vi "ME_acquire_19_DeltaForce_Daq_SteppingMode.vi"() -> ()   [LabVIEW 2015]
doc: "Use this template to build a producer/consumer design pattern. Use this template when you need to execute a process, such as data analysis, when a data source, such as a triggered acquisition, produces data at an uneven rate and you need to execute the process when the data becomes available."
uses:
  Mode.ctl
  oxford_driver/Oxford Drivers/BUSGEN.LLB/OxfordAddress.ctl
  <vilib>/Analysis/baseanly.llb/Mean (DBL).vi
  <vilib>/DAQmx/read.llb/DAQmx Read (Analog 1D DBL 1Chan NSamp).vi
  <vilib>/DAQmx/create/channels.llb/DAQmx Create Channel (AI-Voltage-Basic).vi
  <vilib>/DAQmx/configure/timing.llb/DAQmx Timing (Sample Clock).vi
  <vilib>/Utility/file.llb/Write Delimited Spreadsheet (DBL).vi
  <vilib>/DAQmx/miscellaneous.llb/DAQmx Fill In Error Info.vi
  <vilib>/express/express arith-compare/Formula/XNode/ExpressFormulaBlockNode.xnode
  <vilib>/Analysis/NI_AALBase.lvlib
panel:
  out "fractional index or x":dbl
  out "Stepped P(B)":dbl[][](array[numeric])
  out "TimeUp":bool
  out "meanPolarization":dbl format="%0.2f"
  out "Polarization array":dbl[](array[numeric])
  in  "First Offset?":bool
  out "Last2":dbl
  out "Actual2":dbl
  out "Up/Down":bool
  out "T array":dbl[](array[numeric])
  out "Averaged I(T)":dbl[][](array[numeric])
  in  "Averaged P(T)":dbl[][](array[numeric])
  out "remaining elements 2":T1(array[cluster])
  out "Actual mean":dbl format="%0.6f"
  in  "Averaged dt":dbl[][](array[numeric])
  in  "Averaged P(B)":dbl[][](array[numeric])
  out "LockInR":dbl
  out "deltaUaux":dbl
  out "Actual Voltage (V)":dbl caption="Actual AuxV" step=0.1
  in  "Stop":bool
  out "SaveSweep":bool=TRUE
  out "Measurement File_dn":path
  out "Measurement File_up":path
  out "Measurement File_average":path
  out "Actual Polarization":dbl
  in  "Reset IB?":bool
  in  "First?":bool
  in  "Save Period":dbl=1.0
  out "Averaged I(B)":dbl[][](array[numeric])
  out "P(uC/mm^2)":dbl[](array[numeric])
  in  "Sweep":bool
  out "Offset array":dbl[](array[numeric])
  in  "stop 2":bool
  in  "dB":dbl=0.005
  out "appended array":dbl[][](array[numeric])
  out "Actual B Field (T)":dbl
  out "Actual Temperature (K)":dbl
  out "Actual Current (pA)":dbl
  in  "Tab Control":T2(tab)
  in  "dt (K)":dbl=0.1
  in  "Max temperature (K)":dbl=20.0
  in  "Min Temperature (K)":dbl=4.5
  out "P(T)":cluster{dbl[], dbl[]}[](graph)
  out "I(T)":cluster{dbl[], dbl[]}[](graph)
  in  "Set temperature (K)":dbl=4.5
  in  "Temp Ramping Rate (K/min)":dbl=10.0
  in  "Heater Range":enum16{"Off", "Low", "Medium", "High"}(ring)
  in  "Heater On/Off":bool
  out "Setpoint Temperature (K)":dbl
  out "I(T) /Averaged/":cluster{"B array":dbl[], dbl[]}[](graph)
  out "P(T) /Averaged/":cluster{"B array":dbl[], dbl[]}[](graph)
  in  "Stabilization Time (s)":dbl=5.0
  out "I(B) 3":cluster{dbl[], dbl[]}[](graph)
  out "I(B) /Averaged/":cluster{"B array":dbl[], dbl[]}[](graph)
  out "P(B) /Averaged/":cluster{"B array":dbl[], dbl[]}[](graph)
  out "P(B)":cluster{"yi":dbl[], dbl[]}(graph)
  in  "Set Field (T)":dbl
  in  "Go to Set":bool
  in  "Sweep Rate (T/min)":dbl=2.0 format="%.6f"
  in  "Field To Zero":bool
  out "Target Field":dbl
  in  "Min Field (T)":dbl
  in  "Max Field (T)":dbl=0.15
  in  "Threshold B (T)":dbl
  in  "ReOffset":bool=TRUE
  in  "Window (s)":dbl=6.0
  in  "Field Step (T)":dbl=0.01
  in  "Stepping Mode":bool=TRUE
  out "Ready2Step":bool
  in  "Dwell Time (s)":dbl=1.0
  out "B(t)":dbl(graph)
  out "I(t)":dbl(graph)
  out "P(t)":dbl(graph)
  in  "Max count array":i32[](array[numeric])=[2]
  in  "Magnetic Field array (T)":dbl[](array[numeric])=[0.025, 0.05, 0.075, 0.1, 0.125, 0.15, 0.175, 0.2, 0.225, 0.25, 0.275, 0.3]
  in  "T Sweep Rate Array":dbl[](array[numeric])=[10.0, 20.0]
  in  "secs to wait":dbl=180.0
  out "Wait (s)":dbl
  in  "Directory":string
  out "Finished":bool=TRUE
  out "Step Rate":bool
  out "New":bool=TRUE
  in  "Temperature Array":dbl[](array[numeric])=[4.5, 5.0, 6.0, 7.0, 8.0, 9.0, 10.0, 11.0, 12.0]
  in  "Sweep Rate Array":dbl[](array[numeric])=[2.0, 1.0, 0.5, 0.1, 0.05, 9.0, 10.0, 11.0, 12.0]
  in  "Record ALL":bool
  in  "Max Countl":i32
  out "i":i32
  out "j":i32
  out "Step Temp":bool
  in  "FileName":string
  in  "Measure Noise":bool
  in  "Cycles":i32
  in  "maximum value":dbl=10.0 format="%0.2f"
  in  "minimum value":dbl=-10.0 format="%0.2f"
  in  "physical channels":tag="Dev1/ai1"
  out "PSD (pA/Hz^1/2) Peaks Removed":cluster{"f0":dbl, "df":dbl, "magnitude":dbl[]}(graph)
  out "PSD (pA/Hz^1/2)":cluster{"f0":dbl, "df":dbl, "magnitude":dbl[]}(graph)
  out "Current (pA) Filtered":waveform(dbl)(graph)
  out "Current (pA)":dbl[](graph)
  in  "Samples per channel":i32=1000
  in  "Rate":dbl=1000.0 format="%0.2f"
  in  "Cut-Off Frequency":dbl=100.0 caption="Lower Cut-Off"
  in  "Filter On":bool
  in  "Count":i32=60
  in  "Keithley (IV conv) averaging":i32=10
  in  "Lock_in_Amplifier":refnum<visa-resource-name>="GPIB0::5::INSTR"
  out "Dc offset":dbl
  in  "Calibrate":bool
  in  "IV converter":refnum<visa-resource-name>="GPIB0::20::INSTR"
  in  "Magnetic Field":refnum<visa-resource-name>="GPIB0::21::INSTR"
  out "Time Lag":dbl=0.0500025749206543
  in  "Lake Shore":refnum<visa-resource-name>="GPIB0::11::INSTR"
  in  "Temp Refresh (s)":dbl=0.1
  in  "Sampling rate (Hz)":dbl=10.0
  in  "Gain (V/A)":dbl=1000000000.0
  in  "Sample area (mm^2)":dbl=1.0
  out "B_V":cluster{dbl[], "Best Linear Fit":dbl[]}[](graph)=[{[-0.00769241141, -0.00768011662, -0.0029394633, 0.00271952438, 0.00937200583, 0.0154641889, 0.0217080684, 0.0281692221, 0.0344763397, 0.0407091529, 0.0473661569, 0.0541476438, 0.0611164384, 0.0676637725, 0.073937413, 0.0801511723, 0.0863882257, 0.0933787866, 0.0997676928, 0.106163316, 0.113953626, 0.118979018, 0.126030157, 0.132855724, 0.13883398, 0.14631074, 0.153030676, 0.159156864, 0.165801088, 0.17248087, 0.178555009, 0.185285367, 0.192834407, 0.198751051, 0.205413053, 0.212847389, 0.219477697, 0.225574642, 0.232225854, 0.239015189, 0.245675966, 0.252411162, 0.258453848, 0.265211852, 0.271251534, 0.277801221, 0.284008329, 0.291402813, 0.297970768, 0.304082546, 0.310761405, 0.317366634, 0.323522001, 0.330123184, 0.336841279, 0.343557963, 0.349608435, 0.356238003, 0.363590921, 0.370338319, 0.376962983], "Best Linear Fit"=[0.0, 0.0015, 0.0035, 0.0056, 0.0076, 0.0096, 0.0116, 0.0136, 0.0156, 0.0177, 0.0197, 0.0219, 0.0239, 0.0259, 0.0279, 0.0299, 0.032, 0.034, 0.036, 0.038, 0.04, 0.042, 0.0441, 0.046, 0.048, 0.05, 0.052, 0.054, 0.056, 0.058, 0.06, 0.0621, 0.0643, 0.0663, 0.0684, 0.0704, 0.0725, 0.0745, 0.0765, 0.0787, 0.0807, 0.0827, 0.0847, 0.0868, 0.0888, 0.0908, 0.0928, 0.0948, 0.0968, 0.0988, 0.1008, 0.1028, 0.1048, 0.1069, 0.1091, 0.1111, 0.1131, 0.1152, 0.1173, 0.1193, 0.1213]}, {[-0.00769241141, -0.00768011662, -0.0029394633, 0.00271952438, 0.00937200583, 0.0154641889, 0.0217080684, 0.0281692221, 0.0344763397, 0.0407091529, 0.0473661569, 0.0541476438, 0.0611164384, 0.0676637725, 0.073937413, 0.0801511723, 0.0863882257, 0.0933787866, 0.0997676928, 0.106163316, 0.113953626, 0.118979018, 0.126030157, 0.132855724, 0.13883398, 0.14631074, 0.153030676, 0.159156864, 0.165801088, 0.17248087, 0.178555009, 0.185285367, 0.192834407, 0.198751051, 0.205413053, 0.212847389, 0.219477697, 0.225574642, 0.232225854, 0.239015189, 0.245675966, 0.252411162, 0.258453848, 0.265211852, 0.271251534, 0.277801221, 0.284008329, 0.291402813, 0.297970768, 0.304082546, 0.310761405, 0.317366634, 0.323522001, 0.330123184, 0.336841279, 0.343557963, 0.349608435, 0.356238003, 0.363590921, 0.370338319, 0.376962983], "Best Linear Fit"=[0.002353460844818253, 0.002357267374965663, 0.003824997997530172, 0.005577049655813272, 0.007636692089275871, 0.009522863265806463, 0.01145600043639222, 0.013456406815525209, 0.015409122826751182, 0.01733883381400479, 0.019399876452181594, 0.021499459635718428, 0.023657034245452215, 0.025684122519169482, 0.027626473848249778, 0.02955028565017564, 0.03148130942513291, 0.03364562299316916, 0.03562366117513693, 0.037603778974812686, 0.040015698972850115, 0.04157158615356273, 0.04375465501257369, 0.04586788562152819, 0.0477187843918964, 0.050033627699098075, 0.05211415440778254, 0.05401085368533849, 0.056067939569859164, 0.05813603439385595, 0.06001661903361471, 0.06210037244704129, 0.06443759401357516, 0.0662694173922171, 0.06833200743687069, 0.07063371605572277, 0.07268649347515121, 0.0745741389696738, 0.07663338837489471, 0.07873540137051047, 0.08079761214887074, 0.08288286343195213, 0.08475371006132383, 0.08684602281837933, 0.08871593939391825, 0.09074375613756333, 0.09266550866283872, 0.09495487889775463, 0.09698835150804998, 0.09888058937557581, 0.10094839843403076, 0.10299341126621803, 0.10489914451207855, 0.10694290468187984, 0.10902286140750632, 0.11110238128028392, 0.11297563849525552, 0.11502818680688229, 0.1173046879946565, 0.11939371707962458, 0.12144474708765744]}]
  out "V_I":cluster{dbl[], "Best Linear Fit":dbl[]}[](graph)=[{[0.0, 0.012, 0.026, 0.04, 0.054, 0.068, 0.081, 0.096, 0.11, 0.124, 0.138, 0.153, 0.167, 0.18, 0.195, 0.208, 0.223, 0.236, 0.251, 0.265, 0.279, 0.292, 0.306, 0.32, 0.334, 0.348, 0.362, 0.375, 0.389, 0.403, 0.417, 0.432, 0.446, 0.46, 0.475, 0.489, 0.504, 0.517, 0.531, 0.546, 0.56, 0.574, 0.588, 0.602, 0.616, 0.63, 0.644, 0.658, 0.672, 0.685, 0.699, 0.713, 0.727, 0.742, 0.755, 0.77, 0.784, 0.799, 0.814, 0.827, 0.841], "Best Linear Fit"=[-0.00769241141, -0.00768011662, -0.0029394633, 0.00271952438, 0.00937200583, 0.0154641889, 0.0217080684, 0.0281692221, 0.0344763397, 0.0407091529, 0.0473661569, 0.0541476438, 0.0611164384, 0.0676637725, 0.073937413, 0.0801511723, 0.0863882257, 0.0933787866, 0.0997676928, 0.106163316, 0.113953626, 0.118979018, 0.126030157, 0.132855724, 0.13883398, 0.14631074, 0.153030676, 0.159156864, 0.165801088, 0.17248087, 0.178555009, 0.185285367, 0.192834407, 0.198751051, 0.205413053, 0.212847389, 0.219477697, 0.225574642, 0.232225854, 0.239015189, 0.245675966, 0.252411162, 0.258453848, 0.265211852, 0.271251534, 0.277801221, 0.284008329, 0.291402813, 0.297970768, 0.304082546, 0.310761405, 0.317366634, 0.323522001, 0.330123184, 0.336841279, 0.343557963, 0.349608435, 0.356238003, 0.363590921, 0.370338319, 0.376962983]}, {[0.0, 0.012, 0.026, 0.04, 0.054, 0.068, 0.081, 0.096, 0.11, 0.124, 0.138, 0.153, 0.167, 0.18, 0.195, 0.208, 0.223, 0.236, 0.251, 0.265, 0.279, 0.292, 0.306, 0.32, 0.334, 0.348, 0.362, 0.375, 0.389, 0.403, 0.417, 0.432, 0.446, 0.46, 0.475, 0.489, 0.504, 0.517, 0.531, 0.546, 0.56, 0.574, 0.588, 0.602, 0.616, 0.63, 0.644, 0.658, 0.672, 0.685, 0.699, 0.713, 0.727, 0.742, 0.755, 0.77, 0.784, 0.799, 0.814, 0.827, 0.841], "Best Linear Fit"=[-0.015941127780698654, -0.010342478990544012, -0.0038107220686969304, 0.0027210348531501527, 0.009252791774997235, 0.01578454869684432, 0.02184975155284518, 0.028848062540538483, 0.03537981946238557, 0.041911576384232645, 0.048443333306079736, 0.05544164429377303, 0.061973401215620116, 0.06803860407162098, 0.07503691505931429, 0.08110211791531513, 0.08810042890300844, 0.0941656317590093, 0.10116394274670261, 0.1076956996685497, 0.11422745659039678, 0.12029265944639762, 0.1268244163682447, 0.1333561732900918, 0.13988793021193888, 0.14641968713378595, 0.15295144405563305, 0.15901664691163392, 0.165548403833481, 0.1720801607553281, 0.17861191767717516, 0.18561022866486845, 0.19214198558671555, 0.19867374250856262, 0.20567205349625592, 0.212203810418103, 0.2192021214057963, 0.22526732426179719, 0.23179908118364426, 0.23879739217133758, 0.24532914909318465, 0.2518609060150317, 0.2583926629368788, 0.2649244198587259, 0.271456176780573, 0.27798793370242003, 0.28451969062426713, 0.29105144754611423, 0.2975832044679613, 0.3036484073239622, 0.31018016424580924, 0.3167119211676563, 0.3232436780895034, 0.3302419890771967, 0.3363071919331976, 0.3433055029208909, 0.34983725984273795, 0.35683557083043127, 0.36383388181812454, 0.3698990846741254, 0.3764308415959725]}]
  out "B0 (T)":dbl=0.002883352659639724
  out "B/V (T/V)":dbl=0.28933698328911694
  out "I0 (A)":dbl=-0.009969607826625851
  out "V/I (Ohm)":dbl=0.49959372813071373
  in  "Offset?":bool
  in  "Magnet":bool=TRUE
  in  "Ramp":bool=TRUE
  in  "DaQ":bool
  in  "Moving average":i8=10
  in  "Sample Rate":dbl=1000.0
  in  "Number of Samples":i32=100
  in  "Physical Channel":tag="kartya/ai0"
  in  "Min Voltage":dbl=-5.0
  in  "Max Voltage":dbl=5.0
  in  "Terminal Configuration":i32(ring)=-1 items=["default"=-1, "RSE"=10083, "NRSE"=10078, "Differential"=10106, "Pseudodifferential"=12529]
  out "Confirm":bool
  in  "Dwell Time (ms)":u32=1000
  in  "TimeLag?":bool
  in  "Temp/Magnetic Field":bool
  out "index":i8
  out "Read?":bool
  out "Magnetic Field (T)":dbl[](array[numeric])
  out "Reset":bool
  out "Measured Current (pA)":dbl[](array[numeric])
  out "Elapsed Time (s)":dbl[](array[numeric])
  out "Start time":timestamp
  in  "Enum":T3=enum."Process"
  out "B array":dbl[](array[numeric])
  in  "dB (T)":dbl=0.0025
  in  "Counter":i8
  out "L magnet (H)":dbl
  out "R magnet (mOhm)":dbl
  out "Actual Current (R0)":dbl
  out "Actual Field (T)":dbl
  out "Temperature array":dbl[](array[numeric])
  in  "New Measurement File":bool
  out "Measurement File":path
  out "refnum out":refnum<file>
  in  "Measuring":bool
  in  "Measure /Pause":bool
  in  "stop":bool
  # "DeltaForce"
  # "Discrete"
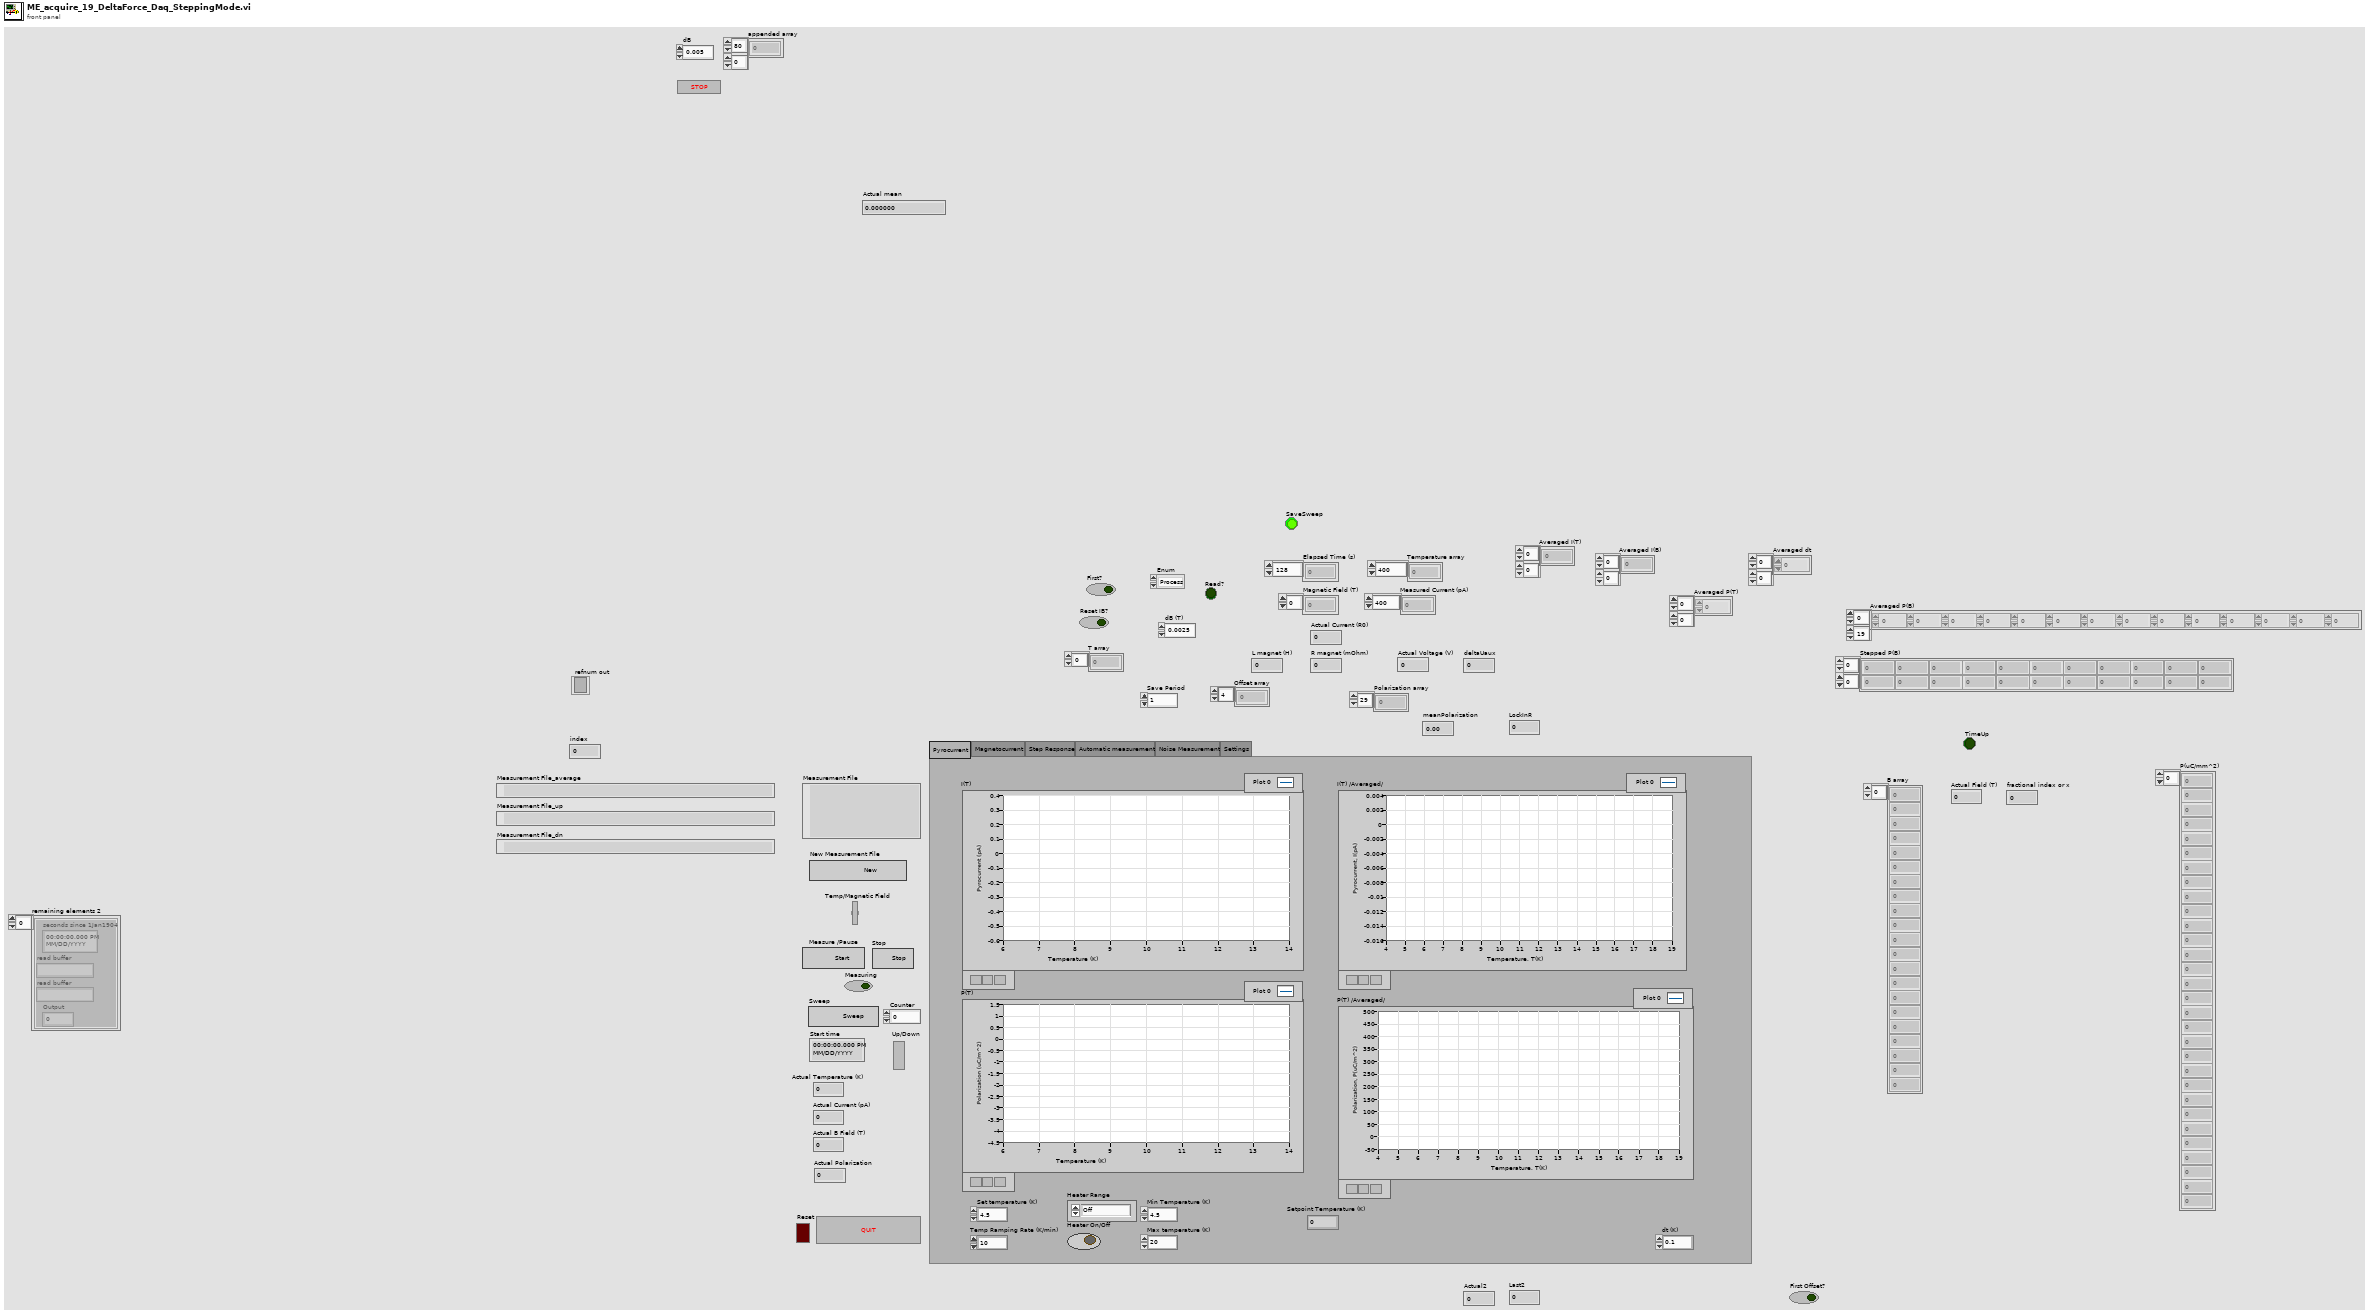
[diagram p1: front panel]
types:
  T1 = cluster{"seconds since 1Jan1904":timestamp, "read buffer":string, "read buffer":string, "Output":dbl}[]
  T2 = enum32{"Pyrocurrent", "Magnetocurrent", "Step Response", "Automatic measurement", "Noise Measurement", "Settings"}
  T3 = typedef "Mode.ctl" = enum16{"Offset", "Process", "Sweep", "StepOxford", "StepDelta", "Plot", "Save", "New", "Return", ""}
  T4 = cluster{"seconds since 1Jan1904":timestamp, "read buffer":string, "read buffer":string, "Output":dbl}
  T5 = enum16{"open", "replace", "create", "open or create", "replace or create", "replace or create with confirmation"}
  T6 = typedef "OxfordAddress.ctl" = cluster{"Com Port":i32, "ISOBUS Address":i32, "GPIB Address":i16, "Communication":enum16{"RS232", "ISOBUS", "GPIB", "Gateway"}}
  T7 = cluster{"B array":dbl[], "Averaged P(B) Out":dbl[]}
  T8 = cluster{"B array":dbl[], "BaselineSubtracted I(B)":dbl[]}
  T9 = cluster{"B array":dbl[], "Averaged P(B) Out":dbl[]}[]
  T10 = cluster{"B array":dbl[], "BaselineSubtracted I(B)":dbl[]}[]
  T11 = cluster{"B array":dbl[], "Averaged P(B)":dbl[]}[]
  T12 = cluster{"T array":dbl[], "Averaged P(T) Out":dbl[]}
  T13 = cluster{"T array":dbl[], "Averaged I(B) out":dbl[]}
  T14 = cluster{"T array":dbl[], "Averaged P(T) Out":dbl[]}[]
  T15 = cluster{"T array":dbl[], "Averaged I(B) out":dbl[]}[]
  T16 = cluster{"V array out (V)":dbl[], "I array out (A)":dbl[]}
  T17 = cluster{"V array out (V)":dbl[], "Best Linear Fit":dbl[]}
  T18 = cluster{"I array out (A)":dbl[], "B array Out":dbl[]}
  T19 = cluster{"I array out (A)":dbl[], "Best Linear Fit 2":dbl[]}
  T20 = cluster{"V array out (V)":dbl[], "Best Linear Fit":dbl[]}[]
  T21 = cluster{"I array out (A)":dbl[], "Best Linear Fit 2":dbl[]}[]
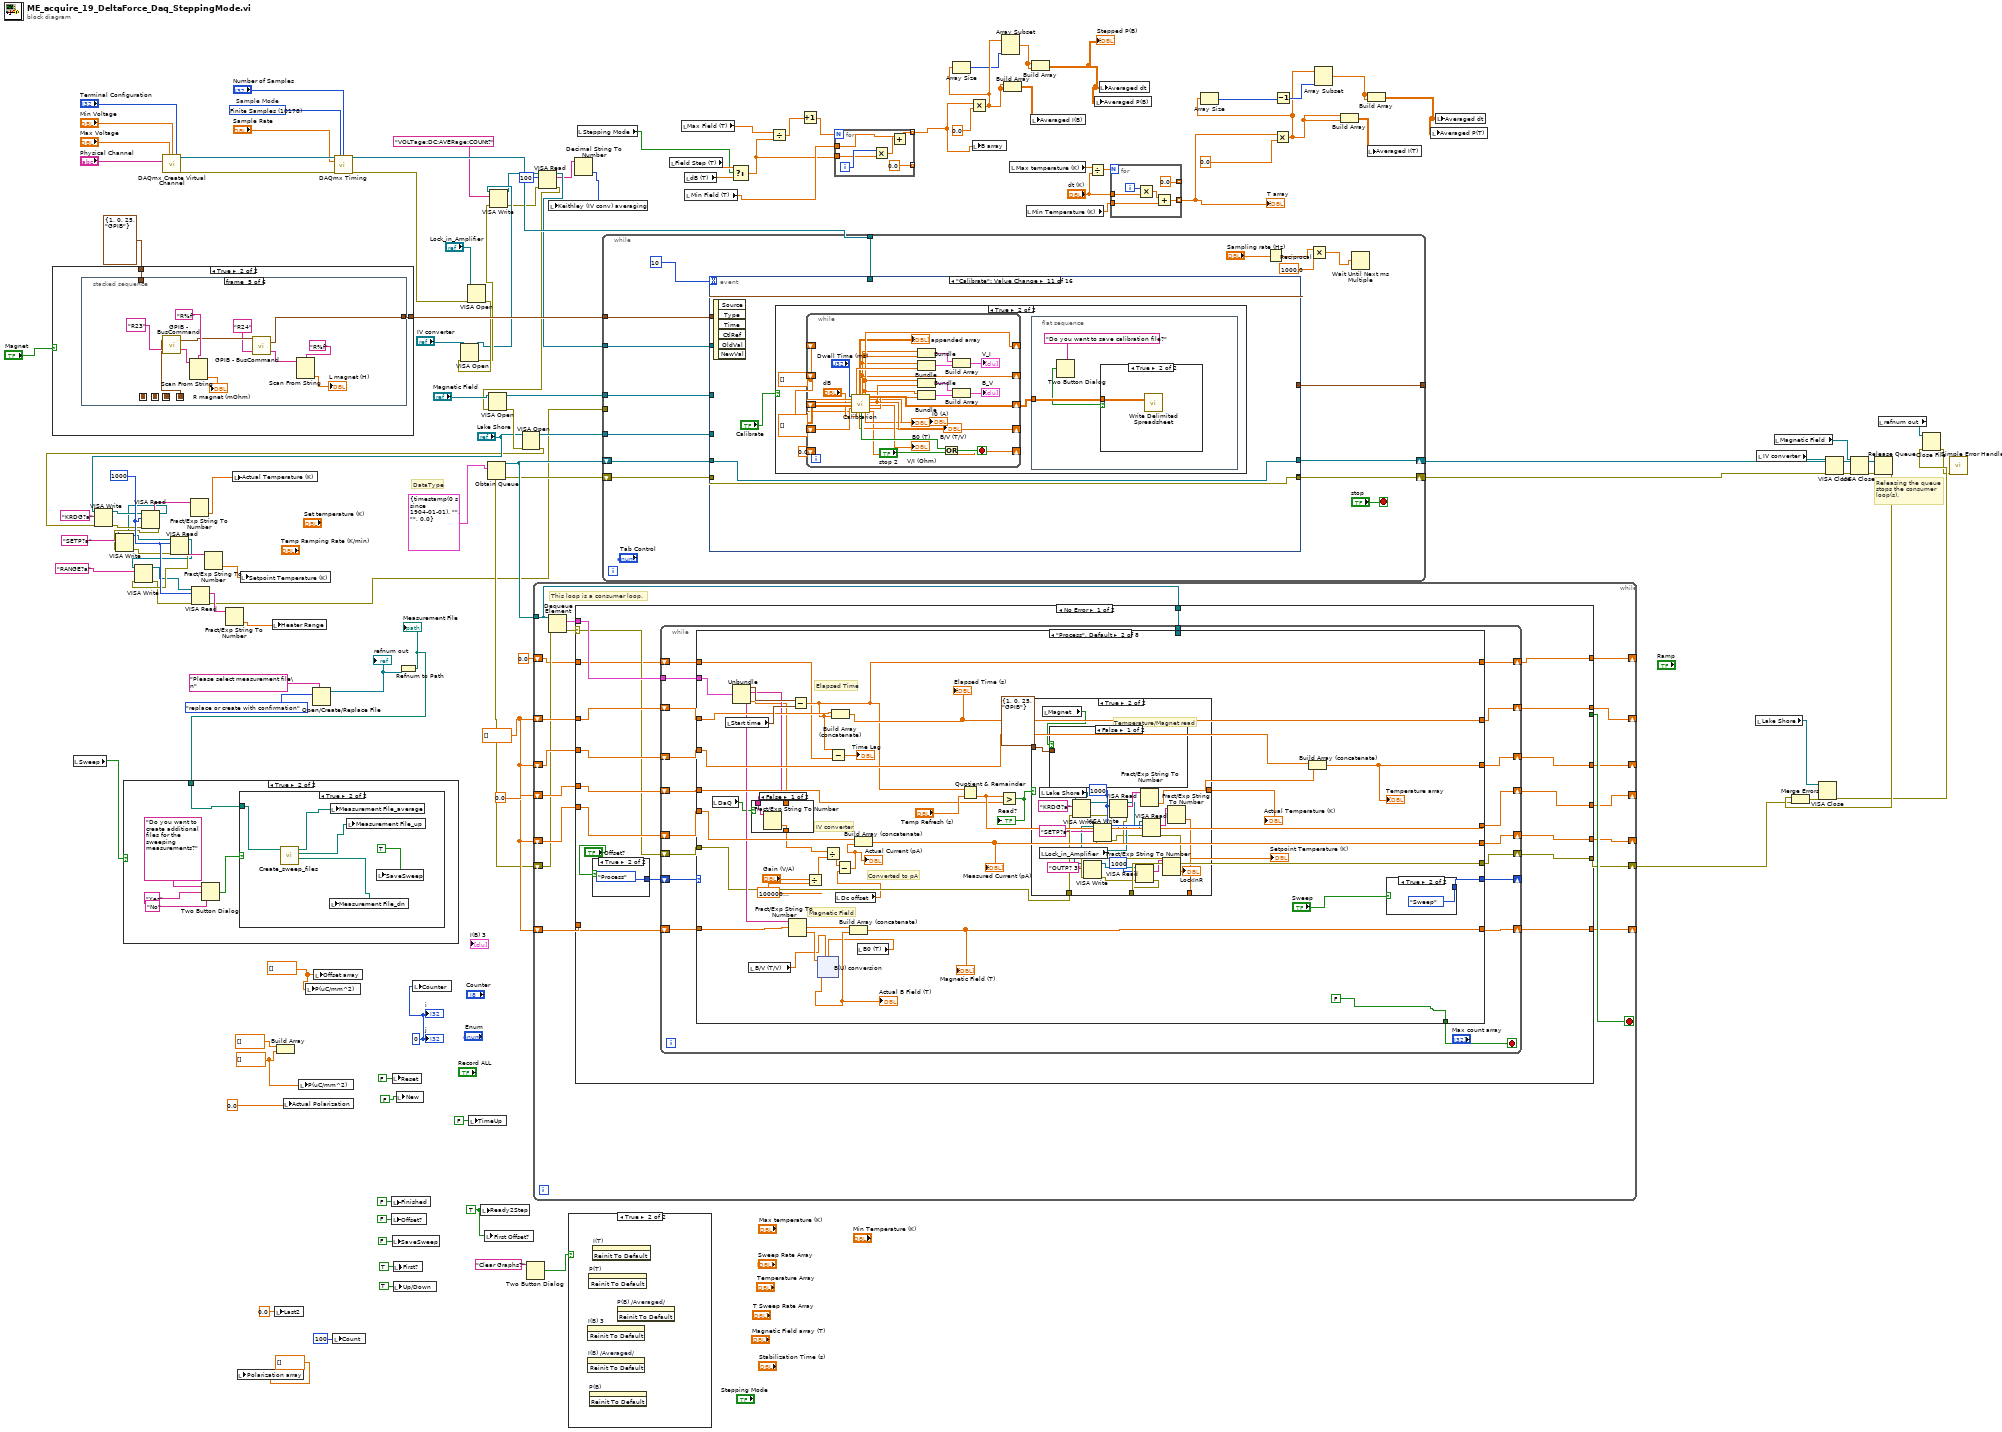
[diagram p0: block diagram]
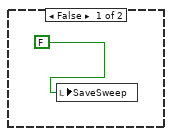
[diagram p4: hidden frame]
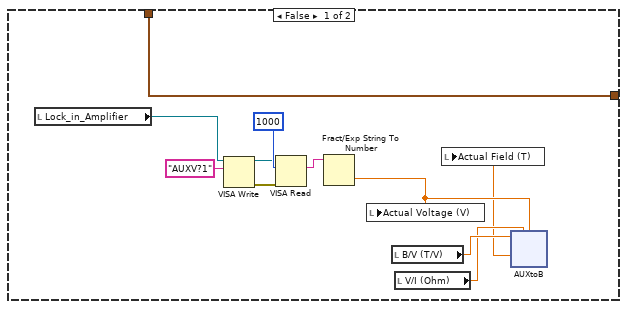
[diagram p5: hidden frame]
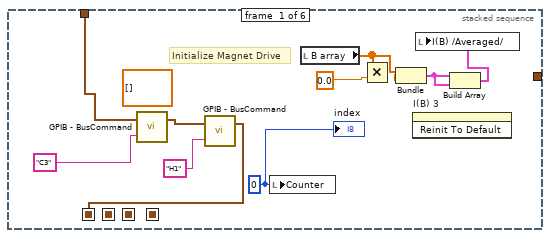
[diagram p6: hidden frame]
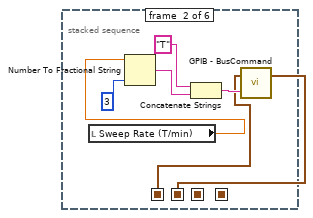
[diagram p7: hidden frame]
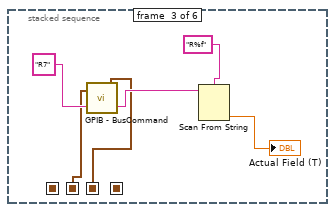
[diagram p8: hidden frame]
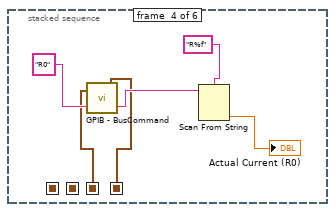
[diagram p9: hidden frame]
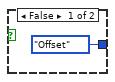
[diagram p11: hidden frame]
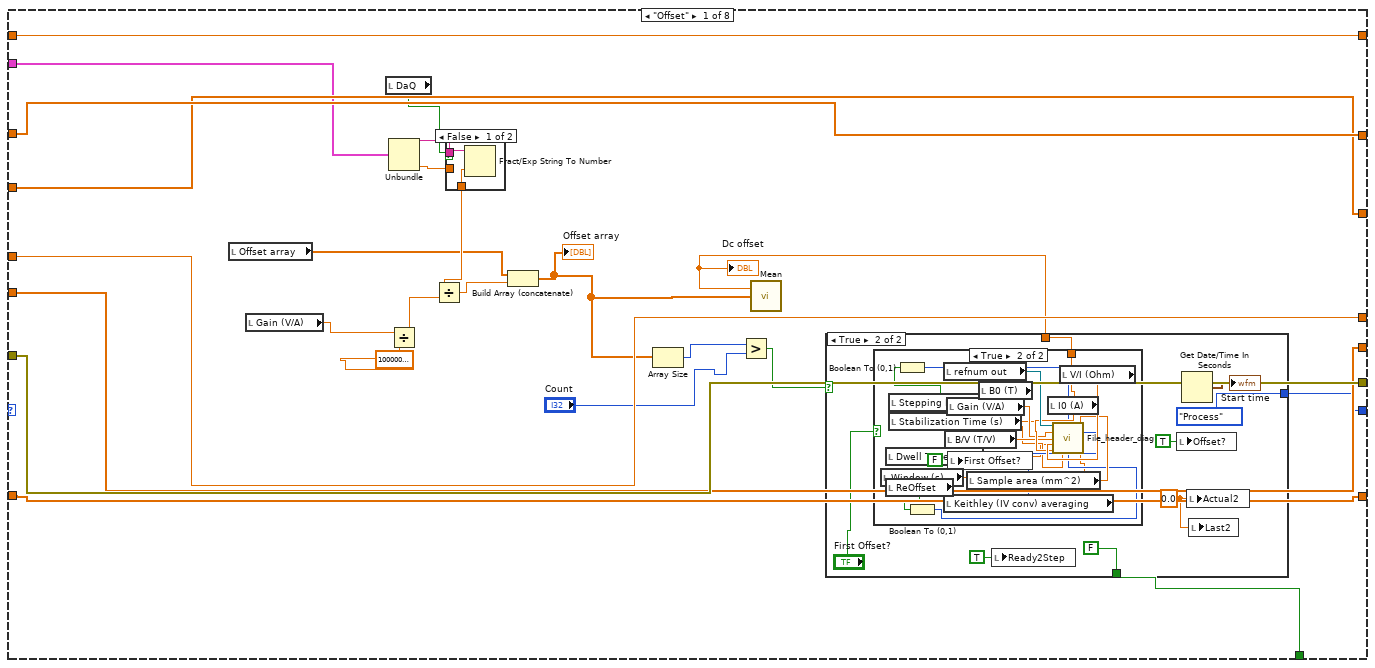
[diagram p12: hidden frame]
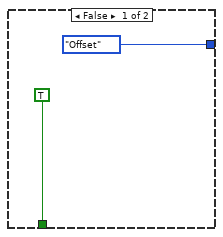
[diagram p14: hidden frame]
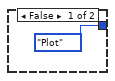
[diagram p17: hidden frame]
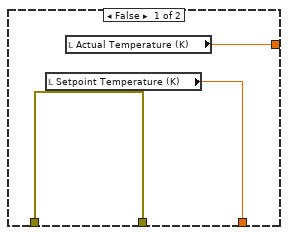
[diagram p18: hidden frame]
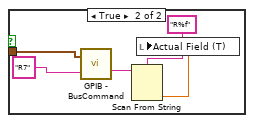
[diagram p19: hidden frame]
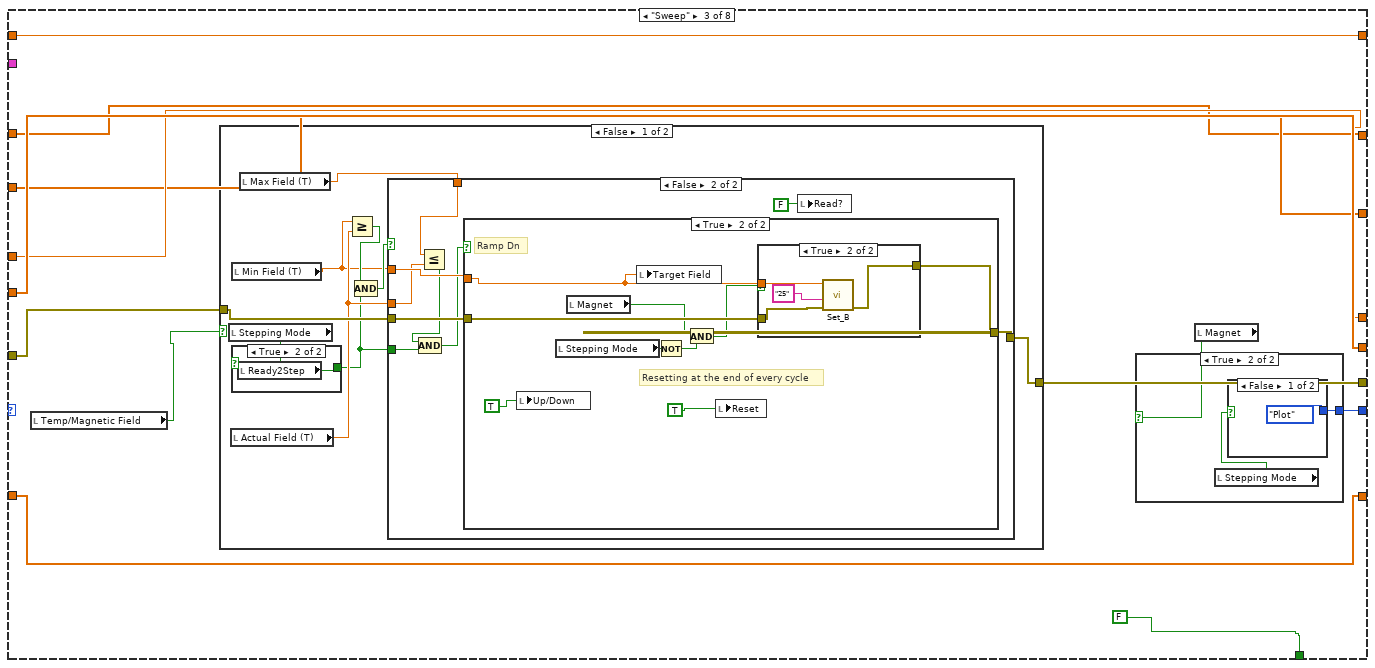
[diagram p20: hidden frame]
diagram:
  w13 = TRUE ("Ready2Step")
  w48 = 10178 items=["Finite Samples"=10178, "Continuous Samples"=10123, "Hardware Timed Single Point"=12522]  # Sample Mode
  w72 = u32 1000 ("byte count")
  w83 = 0 ("j")
  w80 = dbl[] []
  w95 = dbl[] []
  w101 = dbl[] []
  # "DataType"
  # "Releasing the queue stops the consumer loop(s)."
  n1 = case shown="True" "Magnet" {
    tunnel: T6 {"Com Port"=1, "ISOBUS Address"=0, "GPIB Address"=25, "Communication"=enum."GPIB"} ("Address") -> [w135 w149]
    tunnel: [w135 w148] -> w107
    frame False {
      n2 = local read "Lock_in_Amplifier"() -> (w129:refnum<visa-resource-name>)
      n3 = VISA Write(VISA resource name=w129, write buffer="AUXV?1") -> (VISA resource name out=w130:refnum<visa-resource-name>, error out=w134:errorcluster)  [unwired: 1 in, 1 out]
      n4 = VISA Read(VISA resource name=w130, byte count=u32 1000, error in (no error)=w134) -> (read buffer=w133:string)  [unwired: 3 out]
      n5 = Fract/Exp String To Number(string=w133) -> (number=w126:dbl)  [unwired: 3 in, 1 out]
      n6 = local write "Actual Voltage (V)"(w126) -> ()
      n7 = local read "B/V (T/V)"() -> (w128:dbl)
      n8 = local read "V/I (Ohm)"() -> (w127:dbl)
      n9 = xnode "AUXtoB"("BpV"=w128, "Rm"=w127, "Aux"=w126) -> ("Result"=w125:dbl)  [unwired: 1 in, 1 out]
      n10 = local write "Actual Field (T)"(w125) -> ()
    }
    frame True {
      n11 = stacked-sequence {
        seq-local: [w157 _ _ _ _ _] -> [_ w162 _ _ _ _]
        seq-local: [_ w161 _ _ _ _] -> [_ _ w169 _ _ _]
        seq-local: [_ _ w168 _ _ _] -> [_ _ _ w175 _ _]
        seq-local: [_ _ _ w174 _ _] -> [_ _ _ _ w186 _]
        tunnel: w149 -> [w159 _ _ _ _ _]
        tunnel: [_ _ _ _ w184 _] -> w148
        frame #0 {
          (unwired) dbl[][] []
          w155 = i8 0 ("Counter")
          # "Initialize Magnet Drive"
          n12 = call "GPIB - BusCommand.vi"("Command"="C3", "Address"=w159) -> ("Address(thru)"=w158:T6)  [unwired: 1 out]
          n13 = call "GPIB - BusCommand.vi"("Command"="H1", "Address"=w158) -> ("Address(thru)"=w157:T6)  [unwired: 1 out]
          n14 = local write "Counter"(w155) -> ()
          n15 = local read "B array"() -> (w153:dbl[])
          n16 = Multiply(x=w153, y=0.0) -> (x*y=w152:dbl[])
          n17 = Bundle("B array"=w153, w152) -> (w151:cluster{"B array":dbl[], dbl[]})  [unwired: 1 in]
          n18 = invoke on="I(B) 3" class="XYGraph (strict)" method="Reinit To Default"() -> ()  [unwired: 3 in, 3 out]
          n19 = Build Array(w151, w151) -> (w150:cluster{"B array":dbl[], dbl[]}[])
          n20 = local write "I(B) /Averaged/"(w150) -> ()
          "index" <- w155
        }
        frame #1 {
          n21 = local read "Sweep Rate (T/min)"() -> (w163:dbl)
          n22 = Number To Fractional String(number=w163, precision (6)=i16 3) -> (F-format string=w165:string)  [unwired: 2 in]
          n23 = Concatenate Strings("T" ("format string"), w165) -> (w164:string)
          n24 = call "GPIB - BusCommand.vi"("Command"=w164, "Address"=w162) -> ("Address(thru)"=w161:T6)  [unwired: 1 out]
        }
        frame #2 {
          n25 = call "GPIB - BusCommand.vi"("Command"="R7" ("format string"), "Address"=w169) -> ("Reply"=w173:string, "Address(thru)"=w168:T6)
          n26 = Scan From String(format string="R%f" ("remaining string"), input string=w173) -> (output 1=→"Actual Field (T)":dbl)  [unwired: 3 in, 3 out]
        }
        frame #3 {
          n27 = call "GPIB - BusCommand.vi"("Command"="R0" ("format string"), "Address"=w175) -> ("Reply"=w179:string, "Address(thru)"=w174:T6)
          n28 = Scan From String(format string="R%f" ("remaining string"), input string=w179) -> (output 1=→"Actual Current (R0)":dbl)  [unwired: 3 in, 3 out]
        }
        frame #4 {
          n29 = call "GPIB - BusCommand.vi"("Command"="R23" ("format string"), "Address"=w186) -> ("Reply"=w190:string, "Address(thru)"=w185:T6)
          n30 = Scan From String(format string="R%f" ("remaining string"), input string=w190) -> (output 1=→"R magnet (mOhm)":dbl)  [unwired: 3 in, 3 out]
          n31 = call "GPIB - BusCommand.vi"("Command"="R24" ("format string"), "Address"=w185) -> ("Reply"=w182:string, "Address(thru)"=w184:T6)
          n32 = Scan From String(format string="R%f" ("remaining string"), input string=w182) -> (output 1=→"L magnet (H)":dbl)  [unwired: 3 in, 3 out]
        }
        frame #5 {
        }
      }
    }
  }
  n33 = local read "Sweep"() -> (w88:bool)
  n34 = call-poly <vilib>:"DAQmx Create Virtual Channel.vi"("maximum value"="Max Voltage", "minimum value"="Min Voltage", "input terminal configuration"="Terminal Configuration", "physical channels"="Physical Channel") -> ("task out"=w46:refnum<k21>, "error out"=w47:errorcluster)  [unwired: 10 in]
  n35 = local write "Polarization array"(dbl[] [] ("Polarization array")) -> ()
  n36 = local write "Last2"(0.0 ("Last2")) -> ()
  n37 = Build Array(dbl[] [], w80) -> ()  [unwired: 1 out]
  n38 = local write "Actual Polarization"(0.0 ("Actual Polarization")) -> ()
  n39 = local write "P(uC/mm^2)"(w80) -> ()
  n40 = local write "P(uC/mm^2)"(w95) -> ()
  n41 = Open/Create/Replace File(prompt="Please select measurement file\n", operation (0:open)=T5."replace or create with confirmation") -> (refnum out=w104:refnum<file>)  [unwired: 4 in, 2 out]
  "refnum out" <- w104
  n42 = local write "Offset array"(w95) -> ()
  n43 = local write "Count"(100 ("Count")) -> ()
  n44 = call-poly <vilib>:"DAQmx Timing.vi"("task/channels in"=w46, "sample mode"=w48, "samples per channel"="Number of Samples", "rate"="Sample Rate", "error in"=w47) -> ("task out"=w38:refnum<k21>, "error out"=w39:errorcluster)  [unwired: 9 in]
  n45 = local write "Finished"(FALSE ("Finished")) -> ()
  n46 = local write "Offset?"(FALSE ("Offset?")) -> ()
  n47 = local write "Reset"(FALSE ("Reset")) -> ()
  n48 = local write "SaveSweep"(FALSE ("SaveSweep")) -> ()
  n49 = local write "First?"(TRUE ("First?")) -> ()
  n50 = local write "Up/Down"(TRUE ("Up/Down")) -> ()
  n51 = local write "New"(FALSE ("New")) -> ()
  n52 = Refnum to Path(1:w104) -> (0:w87:path)
  "Measurement File" <- w87
  n53 = case shown="True" w88 {
    tunnel: w87 -> [_ w191]
    frame False {
    }
    frame True {
      n54 = Two Button Dialog(message="Do you want to create additional files for the sweeping measurements?" ("string"), 1:"No" ("F button name (\"Cancel\")"), 2:"Yes" ("T button name (\"OK\")")) -> (T button?=w193:bool)
      n55 = case shown="True" w193 {
        tunnel: w191 -> [_ w201]
        frame False {
          n56 = local write "SaveSweep"(FALSE ("SaveSweep")) -> ()
        }
        frame True {
          n57 = call "Create_sweep_files.vi"("Measurement File"=w201) -> ("Path 3"=w198:path, "Path 2"=w199:path, "Path"=w200:path)  [unwired: 8 in]
          n58 = local write "Measurement File_dn"(w198) -> ()
          n59 = local write "Measurement File_average"(w200) -> ()
          n60 = local write "Measurement File_up"(w199) -> ()
          n61 = local write "SaveSweep"(TRUE) -> ()
        }
      }
    }
  }
  n62 = local write "Counter"(w83) -> ()
  n63 = VISA Open(error in (no error)=w39, VISA resource name="Lock_in_Amplifier") -> (error out=w55:errorcluster)  [unwired: 3 in, 1 out]
  n64 = VISA Open(error in (no error)=w55, VISA resource name="IV converter") -> (VISA resource name=w35:refnum<visa-resource-name>, error out=w36:errorcluster)  [unwired: 3 in]
  n65 = local write "TimeUp"(FALSE ("TimeUp")) -> ()
  n66 = local write "Ready2Step"(w13) -> ()
  n67 = local write "First Offset?"(w13) -> ()
  n68 = Obtain Queue(element data type=T4 {"seconds since 1Jan1904"=timestamp(0 s since 1904-01-01), "read buffer"="", "read buffer"="", "Output"=0.0} ("output cluster")) -> (queue out=w124:refnum<queue>, error out=w99:errorcluster)  [unwired: 4 in, 1 out]
  n69 = VISA Write(VISA resource name=w35, write buffer="VOLTage:DC:AVERage:COUNt?", error in (no error)=w36) -> (VISA resource name out=w31:refnum<visa-resource-name>, error out=w33:errorcluster)  [unwired: 1 out]
  n70 = Two Button Dialog(message="Clear Graphs?") -> (T button?=w82:bool)  [unwired: 2 in]
  n71 = while {
    tunnel: w124 -> [w202]
    shift-right: [w215] -> _
    shift-left: w101 -> [w214]
    shift-right: [w213] -> _
    shift-left: w101 -> [w212]
    shift-right: [w211] -> _
    shift-left: w101 -> [w210]
    shift-right: [w209] -> _
    shift-left: 0.0 -> [w208]
    shift-right: [w207] -> _
    shift-left: w101 -> [w206]
    shift-right: [w216] -> w112
    shift-left: w99 -> [w205]
    shift-right: [w204] -> _
    shift-left: 0.0 -> [w203]
    stop <- w217 stop-if-true
    # "This loop is a consumer loop."
    n72 = Dequeue Element(queue=w202, error in (no error)=w205) -> (element=w218:T4, error out=w219:errorcluster)  [unwired: 1 in, 2 out]
    n73 = case shown="No Error" w219 {
      selector: w219 -> [w225 w1221]
      tunnel: w218 -> [w236 _]
      tunnel: [_ TRUE] -> w217
      tunnel: [w224 w1221] -> w216
      tunnel: [w235 w1220] -> w215
      tunnel: w214 -> [w234 w1220]
      tunnel: [w233 w1217] -> w213
      tunnel: w212 -> [w232 w1217]
      tunnel: [w231 w1216] -> w211
      tunnel: w210 -> [w230 w1216]
      tunnel: [w229 w1218] -> w209
      tunnel: w208 -> [w228 w1218]
      tunnel: [w227 w1219] -> w207
      tunnel: w206 -> [w226 w1219]
      tunnel: [w223 w1215] -> w204
      tunnel: w203 -> [w222 w1215]
      tunnel: w202 -> [w220 _]
      frame No Error {
        n74 = case shown="True" "Offset?" {
          tunnel: [Mode."Offset" ("Enum") Mode."Process" ("Enum")] -> w237
          frame False {
          }
          frame True {
          }
        }
        n75 = while {
          shift-right: [w246] -> _
          shift-left: w237 -> [w258]
          tunnel: w236 -> [w257]
          shift-right: [w256] -> w235
          shift-left: w234 -> [w255]
          shift-right: [w248] -> w227
          shift-left: w226 -> [w247]
          shift-right: [w250] -> w229
          shift-left: w228 -> [w249]
          shift-right: [w254] -> w233
          shift-left: w232 -> [w253]
          shift-right: [w244] -> w224
          shift-left: w225 -> [w245]
          shift-right: [w252] -> w231
          shift-left: w230 -> [w251]
          shift-right: [w242] -> w223
          shift-left: w222 -> [w241]
          tunnel: w220 -> [w240]
          stop <- w243 stop-if-true
          n76 = case shown="\"Process\", Default" w258 {
            selector: w258 -> [_ _ _ _ _ _ _ w1208]
            tunnel: w257 -> [w276 w351 _ _ _ _ _ _]
            tunnel: [w282 w348 w409 w558 w702 w820 w984 w1213] -> w256
            tunnel: w255 -> [w282 w341 w409 w558 w702 w816 w984 w1213]
            tunnel: [w277 w347 w412 w555 w704 w822 w982 w1210] -> w254
            tunnel: w253 -> [w277 w346 w412 w555 w704 w817 w982 w1210]
            tunnel: [w278 w345 w414 w554 w699 w823 w980 w1207] -> w252
            tunnel: w251 -> [w278 w344 w414 w554 w699 w818 w980 w1207]
            tunnel: [w280 w340 w411 w556 w700 w826 0.0 w1211] -> w250
            tunnel: w249 -> [w280 w339 w411 w556 w700 w826 _ w1211]
            tunnel: [w281 w336 w410 w557 w701 w821 w983 w1212] -> w248
            tunnel: w247 -> [w281 w337 w410 w557 w701 w819 w983 w1212]
            tunnel: [w266 w334 w407 Mode."Plot" ("Enum") Mode."Save" ("Enum") w827 Mode."Return" ("Enum") w1208] -> w246
            tunnel: w245 -> [w279 w332 w416 w552 w706 w825 w976 w1209]
            tunnel: [w279 w331 w415 w551 w706 w825 w975 w1209] -> w244
            tunnel: [w262 FALSE FALSE FALSE FALSE w814 TRUE TRUE] -> w243
            tunnel: [w265 w328 w408 w549 w703 w824 0.0 w1214] -> w242
            tunnel: w241 -> [w265 w327 w408 w549 w703 w824 _ w1214]
            tunnel: w240 -> [_ _ _ _ _ _ w974 _]
            frame "Offset" {
              n77 = local read "Offset array"() -> (w270:dbl[])
              n78 = local read "Gain (V/A)"() -> (w274:dbl)
              n79 = local read "DaQ"() -> (w261:bool)
              n80 = Unbundle(w276) -> ("read buffer"=w264:string, "Output"=w260:dbl)  [unwired: 2 out]
              n81 = Divide(x=w274, y=1000000000000.0) -> (x/y=w272:dbl)
              n82 = case shown="False" w261 {
                tunnel: [w284 w285] -> w275
                tunnel: w264 -> [w283 _]
                tunnel: w260 -> [_ w285]
                frame False {
                  n83 = Fract/Exp String To Number(string=w283) -> (number=w284:dbl)  [unwired: 3 in, 1 out]
                }
                frame True {
                }
              }
              n84 = Divide(x=w275, y=w272) -> (x/y=w271:dbl)
              n85 = Build Array (concatenate)(w270, w271) -> (w267:dbl[])
              "Offset array" <- w267
              n86 = Array Size(array=w267) -> (size(s)=w269:i32)
              n87 = Greater?(x=w269, y="Count") -> (0:w268:bool)
              n88 = call-poly <vilib>:"Mean.vi"("X"=w267) -> ("mean"=w263:dbl)  [unwired: 1 out]
              "Dc offset" <- w263
              n89 = case shown="True" w268 {
                tunnel: [Mode."Offset" ("Enum") Mode."Process" ("Enum")] -> w266
                tunnel: w263 -> [_ w293]
                tunnel: [TRUE FALSE] -> w262
                frame False {
                }
                frame True {
                  w289 = 0.0 ("Actual2")
                  n90 = case shown="True" "First Offset?" {
                    tunnel: w293 -> [_ w307]
                    frame False {
                    }
                    frame True {
                      n91 = local read "Window (s)"() -> (w297:dbl)
                      n92 = local read "Dwell Time (s)"() -> (w296:dbl)
                      n93 = local read "ReOffset"() -> (w301:bool)
                      n94 = local read "Stepping Mode"() -> (w304:bool)
                      n95 = local read "Stabilization Time (s)"() -> (w298:dbl)
                      n96 = Boolean To (0,1)(Boolean=w304) -> (0, 1=w303:i16)
                      n97 = Boolean To (0,1)(Boolean=w301) -> (0, 1=w300:i16)
                      n98 = local read "refnum out"() -> (w312:refnum<file>)
                      n99 = local read "Keithley (IV conv) averaging"() -> (w306:i32)
                      n100 = local read "B/V (T/V)"() -> (w308:dbl)
                      n101 = local read "Gain (V/A)"() -> (w309:dbl)
                      n102 = local write "First Offset?"(FALSE ("First Offset?")) -> ()
                      n103 = local read "Sample area (mm^2)"() -> (w305:dbl)
                      n104 = local read "B0 (T)"() -> (w299:dbl)
                      n105 = local read "I0 (A)"() -> (w310:dbl)
                      n106 = local read "V/I (Ohm)"() -> (w311:dbl)
                      n107 = call "File_header_diag.vi"("Byte Stream File in"=w312, "B/V"=w308, "SteppingMode"=w303, "OFFSET"=w307, "Sample area"=w305, "Gain"=w309, "Averaging"=w306, "V/I"=w311, "DwellTime"=w296, "I0"=w310, "B0"=w299, "Reoffset"=w300, "Stabilization time"=w298, "Window"=w297) -> ()  [unwired: 2 in]
                    }
                  }
                  n108 = local write "Ready2Step"(TRUE ("Ready2Step")) -> ()
                  n109 = local write "Offset?"(TRUE ("Offset?")) -> ()
                  n110 = Get Date/Time In Seconds() -> (seconds since 1Jan1904=→"Start time":timestamp)
                  n111 = local write "Actual2"(w289) -> ()
                  n112 = local write "Last2"(w289) -> ()
                }
              }
            }
            frame "Process", Default {
              # "Converted to pA"
              # "Magnetic Field"
              # "IV converter"
              # "Elapsed Time"
              n113 = local read "DaQ"() -> (w315:bool)
              n114 = local read "Start time"() -> (w349:timestamp)
              n115 = Unbundle(w351) -> ("seconds since 1Jan1904"=w350:timestamp, "read buffer"=w316:string, "read buffer"=w333:string, "Output"=w313:dbl)
              n116 = local read "B/V (T/V)"() -> (w323:dbl)
              n117 = case shown="False" w315 {
                tunnel: w316 -> [w355 _]
                tunnel: [w354 w356] -> w314
                tunnel: w313 -> [_ w356]
                frame False {
                  n118 = Fract/Exp String To Number(string=w355) -> (number=w354:dbl)  [unwired: 3 in, 1 out]
                }
                frame True {
                }
              }
              n119 = Fract/Exp String To Number(string=w333) -> (number=w343:dbl)  [unwired: 3 in, 1 out]
              n120 = Subtract(x=w350, y=w349) -> (x-y=w328:dbl)
              n121 = Divide(x="Gain (V/A)", y=1000000000000.0) -> (x/y=w326:dbl)
              n122 = Divide(x=w314, y=w326) -> (x/y=w321:dbl)
              n123 = Subtract(x=w328, y=w327) -> (x-y=→"Time Lag":dbl)
              n124 = Build Array (concatenate)(w341, w328) -> (w348:dbl[])
              "Elapsed Time (s)" <- w348
              n125 = local read "Dc offset"() -> (w319:dbl)
              n126 = Subtract(x=w321, y=w319) -> (x-y=w320:dbl)
              "Actual Current (pA)" <- w320
              n127 = Build Array (concatenate)(w346, w320) -> (w347:dbl[])
              "Measured Current (pA)" <- w347
              n128 = local read "B0 (T)"() -> (w322:dbl)
              n129 = xnode "B(U) conversion"("V"=w343, "BpV"=w323, "B0"=w322) -> ("Result"=w342:dbl)  [unwired: 1 in, 1 out]
              "Actual B Field (T)" <- w342
              n130 = Build Array (concatenate)(w344, w342) -> (w345:dbl[])
              "Magnetic Field (T)" <- w345
              n131 = Quotient & Remainder(x=w328, y="Temp Refresh (s)") -> (floor(x/y)=w340:dbl)  [unwired: 1 out]
              n132 = Greater?(x=w340, y=w339) -> (0:w338:bool)
              "Read?" <- w338
              n133 = case shown="True" w338 {
                tunnel: [w360 w385] -> w335
                tunnel: w332 -> [w361 w384]
                tunnel: [w361 w364] -> w331
                tunnel: T6 {"Com Port"=1, "ISOBUS Address"=0, "GPIB Address"=25, "Communication"=enum."GPIB"} ("Address") -> [_ w383]
                tunnel: [w359 w379] -> w317
                frame False {
                  n134 = local read "Setpoint Temperature (K)"() -> (w359:dbl)
                  n135 = local read "Actual Temperature (K)"() -> (w360:dbl)
                }
                frame True {
                  w380 = u32 1000 ("byte count")
                  # "Temperature/Magnet read"
                  n136 = local read "Lock_in_Amplifier"() -> (w368:refnum<visa-resource-name>)
                  n137 = local read "Lake Shore"() -> (w382:refnum<visa-resource-name>)
                  n138 = local read "Magnet"() -> (w371:bool)
                  n139 = case shown="False" w371 {
                    tunnel: w383 -> [_ w389]
                    frame False {
                    }
                    frame True {
                      n140 = call "GPIB - BusCommand.vi"("Command"="R7" ("format string"), "Address"=w389) -> ("Reply"=w390:string)  [unwired: 1 out]
                      n141 = Scan From String(format string="R%f" ("remaining string"), input string=w390) -> (output 1=w388:dbl)  [unwired: 3 in, 3 out]
                      n142 = local write "Actual Field (T)"(w388) -> ()
                    }
                  }
                  n143 = VISA Write(VISA resource name=w382, write buffer="KRDG?a", error in (no error)=w384) -> (VISA resource name out=w378:refnum<visa-resource-name>, error out=w376:errorcluster)  [unwired: 1 out]
                  n144 = VISA Read(VISA resource name=w378, byte count=w380, error in (no error)=w376) -> (VISA resource name out=w377:refnum<visa-resource-name>, read buffer=w386:string, error out=w375:errorcluster)  [unwired: 1 out]
                  n145 = VISA Write(VISA resource name=w377, write buffer="SETP?a", error in (no error)=w375) -> (VISA resource name out=w373:refnum<visa-resource-name>, error out=w374:errorcluster)  [unwired: 1 out]
                  n146 = Fract/Exp String To Number(string=w386) -> (number=w385:dbl)  [unwired: 3 in, 1 out]
                  n147 = VISA Read(VISA resource name=w373, byte count=w380, error in (no error)=w374) -> (read buffer=w372:string, error out=w370:errorcluster)  [unwired: 2 out]
                  n148 = VISA Write(VISA resource name=w368, write buffer="OUTP? 3", error in (no error)=w370) -> (VISA resource name out=w367:refnum<visa-resource-name>, error out=w369:errorcluster)  [unwired: 1 out]
                  n149 = VISA Read(VISA resource name=w367, byte count=u32 1000, error in (no error)=w369) -> (read buffer=w363:string, error out=w364:errorcluster)  [unwired: 2 out]
                  n150 = Fract/Exp String To Number(string=w363) -> (number=→"LockInR":dbl)  [unwired: 3 in, 1 out]
                  n151 = Fract/Exp String To Number(string=w372) -> (number=w379:dbl)  [unwired: 3 in, 1 out]
                }
              }
              "Actual Temperature (K)" <- w335
              "Setpoint Temperature (K)" <- w317
              n152 = Build Array (concatenate)(w337, w335) -> (w336:dbl[])
              "Temperature array" <- w336
              n153 = case shown="True" "Sweep" {
                tunnel: [Mode."Plot" ("Enum") Mode."Sweep" ("Enum")] -> w334
                frame False {
                }
                frame True {
                }
              }
            }
            frame "Sweep" {
              n154 = local read "Temp/Magnetic Field"() -> (w406:bool)
              n155 = case shown="False" w406 {
                tunnel: w416 -> [w429 w496]
                tunnel: [w428 w495] -> w415
                frame False {
                  n156 = local read "Stepping Mode"() -> (w423:bool)
                  n157 = local read "Actual Field (T)"() -> (w425:dbl)
                  n158 = local read "Min Field (T)"() -> (w424:dbl)
                  n159 = case shown="True" w423 {
                    tunnel: [w431 w432] -> w422
                    frame False {
                      n160 = local read "Read?"() -> (w431:bool)
                    }
                    frame True {
                      n161 = local read "Ready2Step"() -> (w432:bool)
                    }
                  }
                  n162 = local read "Max Field (T)"() -> (w430:dbl)
                  n163 = Greater Or Equal?(x=w424, y=w425) -> (x >= y?=w427:bool)
                  n164 = Compound Arithmetic op=AND(w427, w422) -> (w426:bool)
                  n165 = case shown="False" w426 {
                    tunnel: [w435 w476] -> w428
                    tunnel: w430 -> [w433 w475]
                    tunnel: w424 -> [_ w474]
                    tunnel: w425 -> [_ w473]
                    tunnel: w429 -> [w436 w472]
                    tunnel: w422 -> [_ w469]
                    frame True {
                      # "Ramp Up"
                      n166 = case shown="False" "First?" {
                        tunnel: [TRUE ("Save") FALSE ("Save")] -> w439
                        tunnel: [w461 w465] -> w438
                        frame False {
                          n167 = local read "Counter"() -> (w464:i8)
                          n168 = local write "Actual Polarization"(0.0 ("Actual Polarization")) -> ()
                          n169 = Increment(x=w464) -> (x+1=w461:i8)
                          n170 = local write "Counter"(w461) -> ()
                        }
                        frame True {
                          n171 = local read "Counter"() -> (w465:i8)
                          n172 = local write "First?"(FALSE ("First?")) -> ()
                        }
                      }
                      "Reset" <- w439
                      n173 = local write "Read?"(FALSE ("Read?")) -> ()
                      n174 = local read "Record ALL"() -> (w434:bool)
                      n175 = case shown="False" w434 {
                        tunnel: w438 -> [_ w446]
                        tunnel: [FALSE w444] -> w437
                        frame False {
                        }
                        frame True {
                          n176 = Greater?(x=w446, y="Max Countl") -> (0:w444:bool)
                        }
                      }
                      n177 = case shown="False" w437 {
                        tunnel: w436 -> [w453 w460]
                        tunnel: [w452 w460] -> w435
                        tunnel: w433 -> [w451 _]
                        frame False {
                          n178 = local read "Stepping Mode"() -> (w449:bool)
                          n179 = local read "Magnet"() -> (w450:bool)
                          n180 = Not(x=w449) -> (.not. x?=w448:bool)
                          n181 = And(x=w448, y=w450) -> (x .and. y?=w447:bool)
                          n182 = case shown="False" w447 {
                            tunnel: w453 -> [w454 w457]
                            tunnel: [w454 w456] -> w452
                            tunnel: w451 -> [_ w455]
                            frame False {
                            }
                            frame True {
                              n183 = call "Set_B.vi"("error in (no error)"=w457, "address string"="25", "Set Field (T)"=w455) -> ("error out"=w456:errorcluster)  [unwired: 8 in]
                            }
                          }
                          "Target Field" <- w451
                        }
                        frame True {
                          "New" <- TRUE
                        }
                      }
                      "Up/Down" <- FALSE ("Up/Down")
                    }
                    frame False {
                      n184 = Less Or Equal?(x=w475, y=w473) -> (x <= y?=w470:bool)
                      n185 = Compound Arithmetic op=AND(w470, w469) -> (w468:bool)
                      n186 = case shown="True" w468 {
                        tunnel: [w477 w484] -> w476
                        tunnel: w474 -> [_ w482]
                        tunnel: w472 -> [w477 w485]
                        frame False {
                        }
                        frame True {
                          # "Resetting at the end of every cycle"
                          # "Ramp Dn"
                          n187 = local write "Up/Down"(TRUE ("Up/Down")) -> ()
                          n188 = local read "Stepping Mode"() -> (w481:bool)
                          n189 = local read "Magnet"() -> (w479:bool)
                          n190 = local write "Target Field"(w482) -> ()
                          n191 = Not(x=w481) -> (.not. x?=w480:bool)
                          n192 = And(x=w479, y=w480) -> (x .and. y?=w478:bool)
                          n193 = local write "Reset"(TRUE ("Reset")) -> ()
                          n194 = case shown="True" w478 {
                            tunnel: w485 -> [w487 w490]
                            tunnel: [w487 w489] -> w484
                            tunnel: w482 -> [_ w488]
                            frame False {
                            }
                            frame True {
                              n195 = call "Set_B.vi"("error in (no error)"=w490, "address string"="25", "Set Field (T)"=w488) -> ("error out"=w489:errorcluster)  [unwired: 8 in]
                            }
                          }
                        }
                      }
                      n196 = local write "Read?"(FALSE ("Read?")) -> ()
                    }
                  }
                }
                frame True {
                  n197 = local read "Setpoint Temperature (K)"() -> (w494:dbl)
                  n198 = local read "Min Temperature (K)"() -> (w493:dbl)
                  n199 = local read "Read?"() -> (w499:bool)
                  n200 = local read "Max temperature (K)"() -> (w492:dbl)
                  n201 = Equal?(x=w494, y=w493) -> (x = y?=w497:bool)
                  n202 = And(x=w497, y=w499) -> (x .and. y?=w498:bool)
                  n203 = case shown="False" w498 {
                    tunnel: [w501 w537] -> w495
                    tunnel: w492 -> [w508 w536]
                    tunnel: w493 -> [_ w535]
                    tunnel: w494 -> [_ w533]
                    tunnel: w496 -> [w502 w532]
                    frame True {
                      # "Ramp Up"
                      n204 = local read "First?"() -> (w512:bool)
                      n205 = case shown="False" w512 {
                        tunnel: [TRUE ("Save") FALSE ("Save")] -> w504
                        tunnel: [w524 w530] -> w506
                        frame False {
                          n206 = local read "Counter"() -> (w527:i8)
                          n207 = local write "Actual Polarization"(0.0 ("Actual Polarization")) -> ()
                          n208 = Increment(x=w527) -> (x+1=w524:i8)
                          n209 = local write "Counter"(w524) -> ()
                        }
                        frame True {
                          n210 = local read "Counter"() -> (w530:i8)
                          n211 = local write "First?"(FALSE ("First?")) -> ()
                        }
                      }
                      n212 = local write "Read?"(FALSE ("Read?")) -> ()
                      n213 = local write "Up/Down"(FALSE ("Up/Down")) -> ()
                      n214 = Number To Fractional String(number=w508, precision (6)=i16 3) -> (F-format string=w510:string)  [unwired: 2 in]
                      n215 = local read "Record ALL"() -> (w507:bool)
                      n216 = Concatenate Strings("SETP 1," ("write buffer"), w510) -> (w503:string)
                      n217 = case shown="True" w507 {
                        tunnel: w506 -> [_ w523]
                        tunnel: [FALSE w522] -> w505
                        frame False {
                        }
                        frame True {
                          n218 = local read "Max Countl"() -> (w521:i32)
                          n219 = Greater?(x=w523, y=w521) -> (0:w522:bool)
                        }
                      }
                      n220 = local write "Reset"(w504) -> ()
                      n221 = case shown="True" w505 {
                        tunnel: w503 -> [w517 _]
                        tunnel: w502 -> [w515 w518]
                        tunnel: [w514 w518] -> w501
                        frame False {
                          n222 = local read "Lake Shore"() -> (w516:refnum<visa-resource-name>)
                          n223 = VISA Write(VISA resource name=w516, write buffer=w517, error in (no error)=w515) -> (error out=w514:errorcluster)  [unwired: 2 out]
                        }
                        frame True {
                          n224 = local write "New"(TRUE ("New")) -> ()
                        }
                      }
                    }
                    frame False {
                      n225 = Equal?(x=w536, y=w533) -> (x = y?=w534:bool)
                      n226 = case shown="True" w534 {
                        tunnel: [w538 w542] -> w537
                        tunnel: w535 -> [_ w541]
                        tunnel: w532 -> [w538 w543]
                        frame False {
                        }
                        frame True {
                          w539 = TRUE ("Reset")
                          # "Ramp Dn"
                          n227 = Number To Fractional String(number=w541, precision (6)=i16 3) -> (F-format string=w545:string)  [unwired: 2 in]
                          n228 = local write "Reset"(w539) -> ()
                          n229 = local write "Up/Down"(w539) -> ()
                          n230 = local read "Lake Shore"() -> (w540:refnum<visa-resource-name>)
                          n231 = Concatenate Strings("SETP 1," ("write buffer"), w545) -> (w547:string)
                          n232 = VISA Write(VISA resource name=w540, write buffer=w547, error in (no error)=w543) -> (error out=w542:errorcluster)  [unwired: 2 out]
                        }
                      }
                      n233 = local write "Read?"(FALSE ("Read?")) -> ()
                    }
                  }
                }
              }
              n234 = local read "Magnet"() -> (w405:bool)
              n235 = case shown="True" w405 {
                tunnel: [Mode."StepDelta" ("Enum") w419] -> w407
                frame False {
                }
                frame True {
                  n236 = local read "Stepping Mode"() -> (w418:bool)
                  n237 = case shown="False" w418 {
                    tunnel: [Mode."Plot" ("Enum") Mode."StepDelta" ("Enum")] -> w419
                    frame False {
                    }
                    frame True {
                    }
                  }
                }
              }
            }
            frame "StepDelta" {
              n238 = local read "Stepping Mode"() -> (w550:bool)
              n239 = case shown="True" w550 {
                tunnel: w552 -> [w560 w614]
                tunnel: [w559 w612] -> w551
                tunnel: w549 -> [_ w613]
                frame False {
                  n240 = flat-sequence {
                    tunnel: w560 -> [w569]
                    tunnel: [w568] -> w559
                    tunnel: [Mode."Plot" ("Enum")] -> _
                    frame #0 {
                      # "Check if it is time to step Field"
                      n241 = local read "Sweep Rate (T/min)"() -> (w570:dbl)
                      n242 = local read "B/V (T/V)"() -> (w562:dbl)
                      n243 = local read "Time Lag"() -> (w566:dbl)
                      n244 = xnode "Sweep Delay"("SweepRate"=w570, "Resolution"=0.001 ("Voltage Step (V)"), "BpV"=w562) -> ("Result"=w567:dbl)  [unwired: 1 in, 1 out]
                      n245 = Divide(x=w566, y=w567) -> (x/y=w564:dbl)
                      n246 = Multiply(x=0.001 ("y"), y=w564) -> (x*y=w563:dbl)
                      "deltaUaux" <- w563
                      n247 = stacked-sequence {
                        tunnel: w569 -> [_ w594]
                        tunnel: [_ w593] -> w568
                        tunnel: w563 -> [w572 _]
                        frame #0 {
                          n248 = local read "Actual Voltage (V)"() -> (w577:dbl)
                          n249 = local read "Up/Down"() -> (w578:bool)
                          n250 = Add(x=w577, y=w572) -> (x+y=w574:dbl)
                          n251 = Subtract(x=w577, y=w572) -> (x-y=w573:dbl)
                          n252 = Select(t=w573, s=w578, f=w574) -> (s? t:f=w576:dbl)
                          "Actual Voltage (V)" <- w576
                          n253 = local read "V/I (Ohm)"() -> (w579:dbl)
                          n254 = local read "B/V (T/V)"() -> (w580:dbl)
                          n255 = xnode "AUXtoB"("BpV"=w580, "Rm"=w579, "Aux"=w576) -> ("Result"=w575:dbl)  [unwired: 1 in, 1 out]
                          n256 = local write "Actual Field (T)"(w575) -> ()
                        }
                        frame #1 {
                          n257 = local read "Actual Voltage (V)"() -> (w599:dbl)
                          n258 = local read "Lock_in_Amplifier"() -> (w595:refnum<visa-resource-name>)
                          n259 = Format Into String(w599) -> (resulting string=w598:string)  [unwired: 3 in, 1 out]
                          n260 = Concatenate Strings("AUXV 1,", w598) -> (w596:string)
                          n261 = VISA Write(VISA resource name=w595, write buffer=w596, error in (no error)=w594) -> (error out=w593:errorcluster)  [unwired: 2 out]
                        }
                      }
                    }
                  }
                }
                frame True {
                  n262 = local read "Up/Down"() -> (w615:bool)
                  n263 = local read "Actual Field (T)"() -> (w616:dbl)
                  n264 = stacked-sequence {
                    tunnel: "Field Step (T)" -> [w622 _ _]
                    tunnel: w616 -> [w621 _ _]
                    tunnel: w615 -> [w620 _ w660]
                    tunnel: w614 -> [w619 w638 _]
                    tunnel: [_ w636 _] -> _
                    tunnel: w613 -> [_ w636 _]
                    tunnel: [_ w638 _] -> w612
                    frame #0 {
                      n265 = local read "Ready2Step"() -> (w618:bool)
                      n266 = case shown="True" w618 {
                        tunnel: w622 -> [_ w628]
                        tunnel: w621 -> [_ w629]
                        tunnel: w620 -> [_ w627]
                        tunnel: w619 -> [w623 w626]
                        tunnel: [w623 w625] -> _
                        frame False {
                        }
                        frame True {
                          n267 = Add(x=w629, y=w628) -> (x+y=w631:dbl)
                          n268 = Subtract(x=w629, y=w628) -> (x-y=w630:dbl)
                          n269 = Select(t=w630, s=w627, f=w631) -> (s? t:f=w633:dbl)
                          n270 = call "Set_B.vi"("error in (no error)"=w626, "address string"="25", "Set Field (T)"=w633) -> ("error out"=w625:errorcluster)  [unwired: 8 in]
                          n271 = local write "Ready2Step"(FALSE ("Ready2Step")) -> ()
                        }
                      }
                    }
                    frame #1 {
                      n272 = local read "Stabilization Time (s)"() -> (w635:dbl)
                      n273 = local read "Last2"() -> (w640:dbl)
                      n274 = Quotient & Remainder(x=w636, y="Window (s)") -> (floor(x/y)=w637:dbl)  [unwired: 1 out]
                      "Actual2" <- w637
                      n275 = Greater?(x=w636, y=w635) -> (0:w634:bool)
                      n276 = Greater?(x=w637, y=w640) -> (0:w639:bool)
                      n277 = case shown="True" w639 {
                        tunnel: w637 -> [_ w651]
                        tunnel: w634 -> [w642 _]
                        frame False {
                          (unwired) Mode."Plot" ("Enum")
                          n278 = local read "Actual Current (pA)"() -> (→"I(t)":dbl)
                          n279 = local read "Actual B Field (T)"() -> (→"B(t)":dbl)
                          n280 = local read "Actual Polarization"() -> (w643:dbl)
                          "P(t)" <- w643
                          n281 = case shown="True" w642 {
                            tunnel: w643 -> [_ w646]
                            frame False {
                            }
                            frame True {
                              n282 = local read "Polarization array"() -> (w647:dbl[])
                              n283 = Build Array (concatenate)(w647, w646) -> (→"Polarization array":dbl[])
                            }
                          }
                        }
                        frame True {
                          n284 = case shown="False" "ReOffset" {
                            frame False {
                              "Ready2Step" <- TRUE ("Ready2Step 2")
                            }
                            frame True {
                              n285 = local read "Sampling rate (Hz)"() -> (w654:dbl)
                              n286 = local write "Offset array"(dbl[] []) -> ()
                              n287 = local write "Offset?"(FALSE ("Offset?")) -> ()
                              n288 = Reciprocal(x=w654) -> (1/x=w653:dbl)
                              n289 = Divide(x="Dwell Time (s)", y=w653) -> (x/y=w656:dbl)
                              n290 = local write "Count"(w656) -> ()
                            }
                          }
                          "Last2" <- w651
                          "TimeUp" <- TRUE ("TimeUp")
                        }
                      }
                    }
                    frame #2 {
                      n291 = local read "TimeUp"() -> (w659:bool)
                      n292 = case shown="True" w659 {
                        tunnel: w660 -> [_ w661]
                        frame False {
                        }
                        frame True {
                          n293 = stacked-sequence {
                            tunnel: w661 -> [w669 _]
                            frame #0 {
                              (unwired) 1 ("index")
                              n294 = local read "Polarization array"() -> (w674:dbl[])
                              n295 = local write "TimeUp"(FALSE ("TimeUp")) -> ()
                              n296 = call-poly <vilib>:"Mean.vi"("X"=w674) -> ("mean"=w673:dbl)  [unwired: 1 out]
                              n297 = flat-sequence {
                                tunnel: w673 -> [w675]
                                tunnel: [w675] -> w665
                                frame #0 {
                                n298 = local write "Polarization array"(dbl[] [] ("Polarization array")) -> ()
                                }
                              }
                              n299 = Select(t=1, s=w669, f=0) -> (s? t:f=w668:i32)
                              n300 = local read "Actual Field (T)"() -> (w664:dbl)
                              n301 = local read "Stepped P(B)"() -> (w666:dbl[][])
                              n302 = local read "B array"() -> (w662:dbl[])
                              n303 = Threshold 1D Array(2:w664, 3:w662) -> (0:w663:dbl)  [unwired: 1 in]
                              "fractional index or x" <- w663
                              n304 = Index Array(array=w666, index (row)=w668, index (col)=w663) -> ()  [unwired: 1 out]
                              n305 = Replace Array Subset(array=w666, new element=w665, index (row)=w668, index (col)=w663) -> (w667:dbl[][])
                              n306 = local write "Stepped P(B)"(w667) -> ()
                              "meanPolarization" <- w665
                            }
                            frame #1 {
                              n307 = local read "B array"() -> (w682:dbl[])
                              n308 = local read "Stepped P(B)"() -> (w685:dbl[][])
                              n309 = Index Array(array=w685, index (row)=1) -> (element=w680:dbl[])  [unwired: 1 in]
                              n310 = Index Array(array=w685, index (row)=0) -> (element=w681:dbl[])  [unwired: 1 in]
                              n311 = Bundle("B array"=w682, "Stepped P(B)"=w681) -> (w679:cluster{"B array":dbl[], "Stepped P(B)":dbl[]})  [unwired: 1 in]
                              n312 = Bundle("B array"=w682, "Stepped P(B)"=w680) -> (w678:cluster{"B array":dbl[], "Stepped P(B)":dbl[]})  [unwired: 1 in]
                              n313 = Build Array(w679, w678) -> (w677:cluster{"B array":dbl[], "Stepped P(B)":dbl[]}[])
                              n314 = local write "I(B) /Averaged/"(w677) -> ()
                            }
                          }
                        }
                      }
                    }
                  }
                }
              }
            }
            frame "Plot" {
              # "dI"
              n315 = local read "P(uC/mm^2)"() -> (w692:dbl[])
              n316 = local read "Sampling rate (Hz)"() -> (w690:dbl)
              n317 = local read "Actual Polarization"() -> (w691:dbl)
              n318 = local read "Actual Current (pA)"() -> (w693:dbl)
              n319 = local read "Time Lag"() -> (w688:dbl)
              n320 = Reciprocal(x=w690) -> (1/x=w689:dbl)
              n321 = Select(t=w688, s="TimeLag?", f=w689) -> (s? t:f=w686:dbl)
              n322 = Multiply(x=w693, y=w686) -> (x*y=w697:dbl)
              n323 = Divide(x=w697, y="Sample area (mm^2)") -> (x/y=w696:dbl)
              n324 = Add(x=w696, y=w691) -> (x+y=w695:dbl)
              "Actual Polarization" <- w695
              n325 = local read "Temp/Magnetic Field"() -> (w705:bool)
              n326 = Build Array (concatenate)(w692, w695) -> (→"P(uC/mm^2)":dbl[])
              n327 = case shown="False" w705 {
                tunnel: w703 -> [_ w756]
                tunnel: w700 -> [_ w752]
                tunnel: w695 -> [w712 w753]
                frame False {
                  # "Magnetic Field plotting"
                  n328 = local read "Up/Down"() -> (w717:bool)
                  n329 = case shown="True" w717 {
                    frame True {
                      # "Down"
                      n330 = local read "I(B) 3"() -> (w727:cluster{dbl[], dbl[]}[])
                      n331 = local read "I(B) 3"() -> (w731:cluster{dbl[], dbl[]}[])
                      n332 = Index Array(array=w727, index=1) -> (element=w725:cluster{dbl[], dbl[]})
                      n333 = Unbundle(w725) -> (w724:dbl[], w723:dbl[])
                      n334 = Index Array(array=w731, index=i8 0 ("t")) -> (element=w728:cluster{dbl[], dbl[]})
                      n335 = local read "Actual Current (pA)"() -> (w718:dbl)
                      n336 = local read "Actual B Field (T)"() -> (w720:dbl)
                      n337 = Build Array (concatenate)(w724, w720) -> (w722:dbl[])
                      n338 = Build Array (concatenate)(w723, w718) -> (w721:dbl[])
                      n339 = Bundle(w722, w721) -> (w719:cluster{dbl[], dbl[]})  [unwired: 1 in]
                      n340 = Build Array(w728, w719) -> (w729:cluster{dbl[], dbl[]}[])
                      n341 = local write "I(B) 3"(w729) -> ()
                    }
                    frame False {
                      # "Up"
                      n342 = local read "I(B) 3"() -> (w743:cluster{dbl[], dbl[]}[])
                      n343 = local read "I(B) 3"() -> (w745:cluster{dbl[], dbl[]}[])
                      n344 = Index Array(array=w743, index=0) -> (element=w741:cluster{dbl[], dbl[]})
                      n345 = Unbundle(w741) -> (w740:dbl[], w739:dbl[])
                      n346 = Index Array(array=w745, index=i8 1 ("t")) -> (element=w734:cluster{dbl[], dbl[]})
                      n347 = local read "Actual B Field (T)"() -> (w735:dbl)
                      n348 = Build Array (concatenate)(w740, w735) -> (w738:dbl[])
                      n349 = local read "Actual Current (pA)"() -> (w732:dbl)
                      n350 = Build Array (concatenate)(w739, w732) -> (w737:dbl[])
                      n351 = Bundle(w738, w737) -> (w736:cluster{dbl[], dbl[]})  [unwired: 1 in]
                      n352 = Build Array(w736, w734) -> (w733:cluster{dbl[], dbl[]}[])
                      n353 = local write "I(B) 3"(w733) -> ()
                    }
                  }
                  n354 = local read "Actual B Field (T)"() -> (w714:dbl)
                  n355 = local read "P(B)"() -> (w716:cluster{"yi":dbl[], dbl[]})
                  n356 = Unbundle(w716) -> ("yi"=w715:dbl[], w713:dbl[])
                  n357 = Build Array (concatenate)(w715, w714) -> (w711:dbl[])
                  n358 = Build Array (concatenate)(w713, w712) -> (w710:dbl[])
                  n359 = Bundle(w711, w710) -> (→"P(B)":cluster{dbl[], dbl[]})  [unwired: 1 in]
                }
                frame True {
                  # "Temperature plotting"
                  n360 = local read "Actual Current (pA)"() -> (w755:dbl)
                  n361 = local read "Actual Temperature (K)"() -> (w754:dbl)
                  n362 = local read "Up/Down"() -> (w748:bool)
                  n363 = local read "P(T)"() -> (w749:cluster{dbl[], dbl[]}[])
                  n364 = local read "Sweep"() -> (w751:bool)
                  n365 = local read "I(T)"() -> (w750:cluster{dbl[], dbl[]}[])
                  n366 = case shown="False" w748 {
                    tunnel: w755 -> [w777 w802]
                    tunnel: w754 -> [w773 w798]
                    tunnel: w753 -> [w771 w796]
                    tunnel: w750 -> [w766 w791]
                    tunnel: w749 -> [w761 w788]
                    tunnel: [w762 w789] -> w747
                    tunnel: [w757 w786] -> w746
                    frame True {
                      n367 = Index Array(array=w766, index=1) -> (element=w770:cluster{dbl[], dbl[]})
                      n368 = Index Array(array=w761, index=1) -> (element=w769:cluster{dbl[], dbl[]})
                      n369 = Index Array(array=w761, index=0) -> (element=w758:cluster{dbl[], dbl[]})
                      n370 = Index Array(array=w766, index=0) -> (element=w763:cluster{dbl[], dbl[]})
                      n371 = Unbundle(w769) -> (w774:dbl[], w772:dbl[])
                      n372 = Unbundle(w770) -> (w781:dbl[], w780:dbl[])
                      n373 = Build Array (concatenate)(w774, w773) -> (w775:dbl[])
                      n374 = Build Array (concatenate)(w772, w771) -> (w776:dbl[])
                      n375 = Build Array (concatenate)(w781, w773) -> (w779:dbl[])
                      n376 = Build Array (concatenate)(w780, w777) -> (w778:dbl[])
                      n377 = Bundle(w775, w776) -> (w759:cluster{dbl[], dbl[]})  [unwired: 1 in]
                      n378 = Bundle(w779, w778) -> (w764:cluster{dbl[], dbl[]})  [unwired: 1 in]
                      n379 = Build Array(w758, w759) -> (w757:cluster{dbl[], dbl[]}[])
                      n380 = Build Array(w763, w764) -> (w762:cluster{dbl[], dbl[]}[])
                    }
                    frame False {
                      n381 = Index Array(array=w791, index=0) -> (element=w795:cluster{dbl[], dbl[]})
                      n382 = Index Array(array=w788, index=0) -> (element=w794:cluster{dbl[], dbl[]})
                      n383 = Index Array(array=w788, index=1) -> (element=w782:cluster{dbl[], dbl[]})
                      n384 = Index Array(array=w791, index=1) -> (element=w785:cluster{dbl[], dbl[]})
                      n385 = Unbundle(w794) -> (w799:dbl[], w797:dbl[])
                      n386 = Unbundle(w795) -> (w806:dbl[], w805:dbl[])
                      n387 = Build Array (concatenate)(w799, w798) -> (w800:dbl[])
                      n388 = Build Array (concatenate)(w797, w796) -> (w801:dbl[])
                      n389 = Build Array (concatenate)(w806, w798) -> (w804:dbl[])
                      n390 = Build Array (concatenate)(w805, w802) -> (w803:dbl[])
                      n391 = Bundle(w800, w801) -> (w783:cluster{dbl[], dbl[]})  [unwired: 1 in]
                      n392 = Bundle(w804, w803) -> (w784:cluster{dbl[], dbl[]})  [unwired: 1 in]
                      n393 = Build Array(w783, w782) -> (w786:cluster{dbl[], dbl[]}[])
                      n394 = Build Array(w784, w785) -> (w789:cluster{dbl[], dbl[]}[])
                    }
                  }
                  "I(T)" <- w747
                  "P(T)" <- w746
                  n395 = case shown="False" w751 {
                    tunnel: w756 -> [w811 _]
                    tunnel: w752 -> [w808 _]
                    frame False {
                      n396 = Quotient & Remainder(x=w811, y="Save Period") -> (x-y*floor(x/y)=w807:dbl)  [unwired: 1 out]
                      n397 = Greater?(x=w808, y=w807) -> (0:w809:bool)
                      n398 = case shown="True" w809 {
                        frame False {
                        }
                        frame True {
                          n399 = local write "Reset"(TRUE) -> ()
                        }
                      }
                    }
                    frame True {
                    }
                  }
                }
              }
            }
            frame "Save" {
              n400 = local read "Reset"() -> (w813:bool)
              n401 = case shown="True" w813 {
                tunnel: w818 -> [w835 w837]
                tunnel: [w835 w840] -> w823
                tunnel: w817 -> [w834 w838]
                tunnel: [w834 w840] -> w822
                tunnel: w819 -> [w833 w839]
                tunnel: [w833 w840] -> w821
                tunnel: [w832 w840] -> w820
                tunnel: w816 -> [w832 w836]
                frame False {
                }
                frame True {
                  n402 = stacked-sequence {
                    tunnel: [_ _ w973] -> w840
                    tunnel: w839 -> [_ w941 _]
                    tunnel: w838 -> [w843 w939 _]
                    tunnel: w837 -> [w844 w940 _]
                    tunnel: w836 -> [w842 w938 _]
                    frame #0 {
                      n403 = local read "Temp/Magnetic Field"() -> (w841:bool)
                      n404 = case shown="True" w841 {
                        tunnel: w844 -> [w851 w925]
                        tunnel: w843 -> [w850 w924]
                        tunnel: w842 -> [w848 w915]
                        frame False {
                          n405 = local read "Stepping Mode"() -> (w846:bool)
                          n406 = local read "Up/Down"() -> (w845:bool)
                          n407 = local read "Counter"() -> (w849:i8)
                          n408 = local read "B array"() -> (w847:dbl[])
                          n409 = case shown="True" w846 {
                            tunnel: w851 -> [w879 _]
                            tunnel: w850 -> [w878 _]
                            tunnel: w849 -> [w877 w881]
                            tunnel: w848 -> [w869 _]
                            tunnel: w847 -> [w863 w880]
                            tunnel: w845 -> [w852 w882]
                            frame False {
                              n410 = local read "Averaged I(B)"() -> (w854:dbl[][])
                              n411 = local read "Sample area (mm^2)"() -> (w859:dbl)
                              n412 = call "Average_IBP_curves_baseline.vi"("I in"=w878, "Averaged P(B) In"="Averaged P(B)", "Counter"=w877, "B0"="Threshold B (T)", "Averaged I(B) In"=w854, "t in"=w869, "B in"=w879, "Averaged dt in"="Averaged dt", "Up/Down"=w852, "Sample area(mm^2)"=w859, "B array"=w863) -> ("Averaged dt Out"=w866:dbl[][], "Averaged P(B) Out"=w855:dbl[][], "BaselineSubtracted I(B)"=w853:dbl[][])  [unwired: 1 in, 1 out]
                              "Averaged I(B)" <- w853
                              n413 = Index Array(array=w855, index (row)=0 ("disabled index (col)")) -> (element=w864:dbl[])  [unwired: 1 in]
                              n414 = Index Array(array=w855, index (row)=1 ("disabled index (col)")) -> (element=w865:dbl[])  [unwired: 1 in]
                              n415 = Index Array(array=w853, index (row)=0 ("disabled index (col)")) -> (element=w871:dbl[])  [unwired: 1 in]
                              n416 = Index Array(array=w853, index (row)=1 ("disabled index (col)")) -> (element=w870:dbl[])  [unwired: 1 in]
                              n417 = local write "Averaged dt"(w866) -> ()
                              n418 = Bundle("B array"=w863, "Averaged P(B) Out"=w864) -> (w862:T7)  [unwired: 1 in]
                              n419 = Bundle("B array"=w863, "Averaged P(B) Out"=w865) -> (w861:T7)  [unwired: 1 in]
                              n420 = local write "Averaged P(B)"(w855) -> ()
                              n421 = Bundle("B array"=w863, "BaselineSubtracted I(B)"=w871) -> (w876:T8)  [unwired: 1 in]
                              n422 = Bundle("B array"=w863, "BaselineSubtracted I(B)"=w870) -> (w875:T8)  [unwired: 1 in]
                              n423 = Build Array(w862, w861) -> (→"P(B) /Averaged/":T9)
                              n424 = Build Array(w876, w875) -> (→"I(B) /Averaged/":T10)
                            }
                            frame True {
                              n425 = stacked-sequence {
                                tunnel: w882 -> [w883 _]
                                tunnel: w881 -> [w885 _]
                                tunnel: w880 -> [w884 _]
                                frame #0 {
                                n426 = case shown="False" w883 {
                                tunnel: w885 -> [w887 _]
                                tunnel: w884 -> [w886 _]
                                frame False {
                                n427 = local read "Stepped P(B)"() -> (w890:dbl[][])
                                n428 = local read "Averaged P(B)"() -> (w889:dbl[][])
                                n429 = call "Average_P_step_2.vi"("Averaged P(B) in"=w889, "B array"=w886, "Counter"=w887, "Stepped P(B)"=w890) -> ("Averaged P(B) out"=w888:dbl[][])  [unwired: 7 in]
                                n430 = local write "Averaged P(B)"(w888) -> ()
                                }
                                frame True {
                                }
                                }
                                }
                                frame #1 {
                                n431 = local read "Averaged P(B)"() -> (w899:dbl[][])
                                n432 = local read "B array"() -> (w896:dbl[])
                                n433 = Index Array(array=w899, index (row)=1) -> (element=w894:dbl[])  [unwired: 1 in]
                                n434 = Index Array(array=w899, index (row)=0) -> (element=w895:dbl[])  [unwired: 1 in]
                                n435 = Bundle("B array"=w896, "Averaged P(B)"=w895) -> (w893:cluster{"B array":dbl[], "Averaged P(B)":dbl[]})  [unwired: 1 in]
                                n436 = Bundle("B array"=w896, "Averaged P(B)"=w894) -> (w892:cluster{"B array":dbl[], "Averaged P(B)":dbl[]})  [unwired: 1 in]
                                n437 = Build Array(w893, w892) -> (w891:T11)
                                n438 = local write "P(B) /Averaged/"(w891) -> ()
                                }
                              }
                            }
                          }
                        }
                        frame True {
                          n439 = local read "T array"() -> (w910:dbl[])
                          n440 = local read "Counter"() -> (w923:i8)
                          n441 = local read "Averaged I(T)"() -> (w902:dbl[][])
                          n442 = local read "Up/Down"() -> (w926:bool)
                          n443 = local read "Averaged dt"() -> (w901:dbl[][])
                          n444 = local read "Sample area (mm^2)"() -> (w906:dbl)
                          n445 = call "Average_ITP_curves.vi"("I in"=w924, "Averaged P(T) In"="Averaged P(T)", "Counter"=w923, "Averaged I(T) In"=w902, "t in"=w915, "T in"=w925, "Averaged dt in"=w901, "Up/Down"=w926, "Sample area(mm^2)"=w906, "T array"=w910) -> ("Averaged I(B) out"=w900:dbl[][], "Averaged dt Out"=w913:dbl[][], "Averaged P(T) Out"=w903:dbl[][])  [unwired: 3 in]
                          "Averaged I(T)" <- w900
                          n446 = Index Array(array=w903, index (row)=0 ("disabled index (col)")) -> (element=w911:dbl[])  [unwired: 1 in]
                          n447 = Index Array(array=w903, index (row)=1 ("disabled index (col)")) -> (element=w912:dbl[])  [unwired: 1 in]
                          n448 = Index Array(array=w900, index (row)=0 ("disabled index (col)")) -> (element=w917:dbl[])  [unwired: 1 in]
                          n449 = Index Array(array=w900, index (row)=1 ("disabled index (col)")) -> (element=w916:dbl[])  [unwired: 1 in]
                          n450 = local write "Averaged dt"(w913) -> ()
                          n451 = Bundle("T array"=w910, "Averaged P(T) Out"=w911) -> (w909:T12)  [unwired: 1 in]
                          n452 = Bundle("T array"=w910, "Averaged P(T) Out"=w912) -> (w908:T12)  [unwired: 1 in]
                          n453 = local write "Averaged P(T)"(w903) -> ()
                          n454 = Bundle("T array"=w910, "Averaged I(B) out"=w917) -> (w922:T13)  [unwired: 1 in]
                          n455 = Bundle("T array"=w910, "Averaged I(B) out"=w916) -> (w921:T13)  [unwired: 1 in]
                          n456 = Build Array(w909, w908) -> (→"P(T) /Averaged/":T14)
                          n457 = Build Array(w922, w921) -> (→"I(T) /Averaged/":T15)
                        }
                      }
                    }
                    frame #1 {
                      # "Save and Reset"
                      n458 = local read "Stepping Mode"() -> (w930:bool)
                      n459 = local read "Up/Down"() -> (w928:bool)
                      n460 = case shown="True" w930 {
                        tunnel: w941 -> [w953 w958]
                        tunnel: w940 -> [w952 w957]
                        tunnel: w939 -> [w951 w956]
                        tunnel: w938 -> [w949 w955]
                        tunnel: [w948 w969] -> w932
                        tunnel: w928 -> [_ w965]
                        tunnel: [w948 w954] -> w929
                        frame False {
                          n461 = local read "P(uC/mm^2)"() -> (w950:dbl[])
                          n462 = Build Array(w953, w952, w951, w949, w950) -> (w948:dbl[][])
                        }
                        frame True {
                          n463 = local read "P(uC/mm^2)"() -> (w959:dbl[])
                          n464 = local read "Averaged P(B)"() -> (w966:dbl[][])
                          n465 = local read "Stepped P(B)"() -> (w967:dbl[][])
                          n466 = Select(t=0, s=w965, f=1) -> (s? t:f=w964:i32)
                          n467 = local read "B array"() -> (w968:dbl[])
                          n468 = Build Array(w958, w957, w956, w955, w959) -> (w954:dbl[][])
                          n469 = Index Array(array=w967, index (row)=w964) -> (element=w963:dbl[])  [unwired: 1 in]
                          n470 = Index Array(array=w966, index (row)=w964) -> (element=w962:dbl[])  [unwired: 1 in]
                          n471 = Build Array(w968, w963, w962) -> (w969:dbl[][])
                        }
                      }
                      n472 = case shown="True" w928 {
                        tunnel: [w970 w971] -> w931
                        frame False {
                          n473 = local read "Measurement File_dn"() -> (w970:path)
                        }
                        frame True {
                          n474 = local read "Measurement File_up"() -> (w971:path)
                        }
                      }
                      n475 = local read "Measurement File"() -> (w933:path)
                      n476 = case shown="True" "Reset IB?" {
                        frame False {
                        }
                        frame True {
                          n477 = local read "Up/Down"() -> (w972:bool)
                          n478 = case shown="False" w972 {
                            frame False {
                              n479 = invoke on="I(B) 3" class="XYGraph (strict)" method="Reinit To Default"() -> ()  [unwired: 3 in, 3 out]
                              n480 = invoke on="I(T)" class="XYGraph (strict)" method="Reinit To Default"() -> ()  [unwired: 3 in, 3 out]
                            }
                            frame True {
                            }
                          }
                        }
                      }
                      n481 = local read "Sweep"() -> (w927:bool)
                      n482 = call-poly <vilib>:"Write Delimited Spreadsheet.vi"("file path (dialog if empty)"=w933, "format (%.3f)"="%.5g", "2D data"=w929, "append to file? (F)"=TRUE, "transpose? (F)"=TRUE) -> ()  [unwired: 9 in, 2 out]
                      n483 = case shown="True" w927 {
                        tunnel: w932 -> [_ w947]
                        tunnel: w931 -> [_ w943]
                        frame False {
                        }
                        frame True {
                          n484 = call-poly <vilib>:"Write Delimited Spreadsheet.vi"("file path (dialog if empty)"=w943, "format (%.3f)"="%.5g", "2D data"=w947, "append to file? (F)"=TRUE ("transpose? (F)"), "transpose? (F)"=FALSE ("append to file? (F)")) -> ()  [unwired: 9 in, 2 out]
                        }
                      }
                      n485 = local write "Reset"(FALSE ("Save")) -> ()
                    }
                    frame #2 {
                      w973 = dbl[] []
                      n486 = local write "P(uC/mm^2)"(w973) -> ()
                    }
                  }
                }
              }
              n487 = local read "New"() -> (w815:bool)
              n488 = case shown="False" w815 {
                tunnel: [Mode."Return" ("Enum") Mode."New" ("Enum")] -> w827
                tunnel: [TRUE FALSE] -> w814
                frame False {
                }
                frame True {
                }
              }
            }
            frame "New" {
              n489 = stacked-sequence {
                seq-local: [_ _ _ _ w1121 _ _] -> [_ _ _ _ _ w1138 _]
                seq-local: [_ _ w1058 _ _ _ _] -> [_ _ _ w1094 _ _ _]
                seq-local: [_ _ _ w1093 _ _ _] -> [_ _ _ _ w1119 _ _]
                seq-local: [_ w1013 _ _ _ _ _] -> [_ _ w1052 _ _ _ _]
                tunnel: T6 {"Com Port"=1, "ISOBUS Address"=0, "GPIB Address"=25, "Communication"=enum."GPIB"} ("Address") -> [_ _ w1057 w1099 _ _ _]
                tunnel: w976 -> [_ w1014 _ _ _ w1139 _]
                tunnel: [_ _ _ _ _ w1141 _] -> w975
                tunnel: w974 -> [_ w1017 _ _ _ _ _]
                frame #0 {
                  w1003 = 1 ("index (row)")
                  w1002 = 0 ("index (row)")
                  # "Save averages"
                  n490 = local read "Temp/Magnetic Field"() -> (w986:bool)
                  n491 = case shown="True" w986 {
                    tunnel: [w1010 w1011] -> w1001
                    tunnel: [w1009 w1012] -> w991
                    frame False {
                      n492 = local read "Averaged P(B)"() -> (w1010:dbl[][])
                      n493 = local read "I(B) /Averaged/"() -> (w1009:cluster{"B array":dbl[], dbl[]}[])
                    }
                    frame True {
                      n494 = local read "Averaged P(T)"() -> (w1011:dbl[][])
                      n495 = local read "I(T) /Averaged/"() -> (w1012:cluster{"B array":dbl[], dbl[]}[])
                    }
                  }
                  n496 = local read "Measurement File_average"() -> (w990:path)
                  n497 = local read "Averaged dt"() -> (w999:dbl[][])
                  n498 = Index Array(array=w999, index (row)=w1002) -> (element=w1000:dbl[])  [unwired: 1 in]
                  n499 = Index Array(array=w999, index (row)=w1003) -> (element=w1007:dbl[])  [unwired: 1 in]
                  n500 = Index Array(array=w991, index=1) -> (element=w995:cluster{"B array":dbl[], dbl[]})
                  n501 = Index Array(array=w991, index=0) -> (element=w994:cluster{"B array":dbl[], dbl[]})
                  n502 = Unbundle(w995) -> ("B array"=w1005:dbl[], w1006:dbl[])
                  n503 = Unbundle(w994) -> ("B array"=w996:dbl[], w997:dbl[])
                  n504 = Index Array(array=w1001, index (row)=w1002) -> (element=w1004:dbl[])  [unwired: 1 in]
                  n505 = Index Array(array=w1001, index (row)=w1003) -> (element=w1008:dbl[])  [unwired: 1 in]
                  n506 = Build Array(w996, w997, w1000, w1004, w1005, w1006, w1007, w1008) -> (w998:dbl[][])
                  n507 = call-poly <vilib>:"Write Delimited Spreadsheet.vi"("file path (dialog if empty)"=w990, "format (%.3f)"="%.5g", "2D data"=w998, "append to file? (F)"=TRUE ("transpose? (F)"), "transpose? (F)"=TRUE ("append to file? (F)")) -> ()  [unwired: 9 in, 2 out]
                }
                frame #1 {
                  w1025 = dbl[] []
                  # "Reset Flags"
                  n508 = Get Date/Time In Seconds() -> (seconds since 1Jan1904=w1026:timestamp)
                  n509 = local write "Measuring"(FALSE ("Measuring")) -> ()
                  n510 = local write "Up/Down"(TRUE ("Up/Down")) -> ()
                  n511 = local write "First?"(TRUE ("First?")) -> ()
                  n512 = local write "Offset?"(FALSE ("Offset?")) -> ()
                  n513 = local write "New"(FALSE ("New")) -> ()
                  n514 = local write "P(uC/mm^2)"(w1025) -> ()
                  n515 = local write "Start time"(w1026) -> ()
                  n516 = local write "Offset array"(w1025) -> ()
                  n517 = local write "Actual Polarization"(0.0 ("Actual Polarization")) -> ()
                  n518 = local write "Up/Down"(TRUE ("Up/Down")) -> ()
                  n519 = local read "Temp/Magnetic Field"() -> (w1015:bool)
                  n520 = local write "Reset"(FALSE ("Reset")) -> ()
                  n521 = case shown="False" w1015 {
                    tunnel: w1014 -> [w1031 w1044]
                    tunnel: [w1029 w1044] -> w1013
                    frame True {
                      w1037 = dbl[] []
                      n522 = local read "B array"() -> (w1039:dbl[])
                      n523 = invoke on="I(T)" class="XYGraph (strict)" method="Reinit To Default"() -> ()  [unwired: 3 in, 3 out]
                      n524 = Build Array(w1037, w1037) -> (w1043:dbl[][])
                      n525 = Multiply(x=w1039, y=0.0) -> (x*y=w1040:dbl[])
                      n526 = Bundle("B array"=w1039, w1040) -> (w1041:cluster{"B array":dbl[], dbl[]})  [unwired: 1 in]
                      n527 = local write "Averaged I(T)"(w1043) -> ()
                      n528 = invoke on="P(T)" class="XYGraph (strict)" method="Reinit To Default"() -> ()  [unwired: 3 in, 3 out]
                      n529 = Build Array(w1041, w1041) -> (w1042:cluster{"B array":dbl[], dbl[]}[])
                      n530 = local write "I(T) /Averaged/"(w1042) -> ()
                      n531 = local read "Set temperature (K)"() -> (w1036:dbl)
                      n532 = Number To Fractional String(number=w1036, precision (6)=i16 3) -> (F-format string=w1033:string)  [unwired: 2 in]
                      n533 = local read "Lake Shore"() -> (w1030:refnum<visa-resource-name>)
                      n534 = Concatenate Strings("SETP 1," ("write buffer"), w1033) -> (w1035:string)
                      n535 = VISA Write(VISA resource name=w1030, write buffer=w1035, error in (no error)=w1031) -> (error out=w1029:errorcluster)  [unwired: 2 out]
                    }
                    frame False {
                      w1045 = dbl[] []
                      n536 = local read "B array"() -> (w1047:dbl[])
                      n537 = invoke on="I(B) 3" class="XYGraph (strict)" method="Reinit To Default"() -> ()  [unwired: 3 in, 3 out]
                      n538 = Build Array(w1045, w1045) -> (w1051:dbl[][])
                      n539 = Multiply(x=w1047, y=0.0) -> (x*y=w1048:dbl[])
                      n540 = Bundle("B array"=w1047, w1048) -> (w1049:cluster{"B array":dbl[], dbl[]})  [unwired: 1 in]
                      n541 = local write "Averaged I(B)"(w1051) -> ()
                      n542 = invoke on="P(B)" class="XYGraph (strict)" method="Reinit To Default"() -> ()  [unwired: 3 in, 3 out]
                      n543 = Build Array(w1049, w1049) -> (w1050:cluster{"B array":dbl[], dbl[]}[])
                      n544 = local write "I(B) /Averaged/"(w1050) -> ()
                    }
                  }
                  n545 = local write "Counter"(i8 0 ("Counter")) -> ()
                  n546 = Flush Queue(queue=w1017) -> (remaining elements=→"remaining elements 2":T1)  [unwired: 1 in, 2 out]
                }
                frame #2 {
                  # "Step"
                  n547 = local read "Sweep Rate Array"() -> (w1055:dbl[])
                  n548 = local read "T Sweep Rate Array"() -> (w1056:dbl[])
                  n549 = local read "Temp/Magnetic Field"() -> (w1053:bool)
                  n550 = local read "j"() -> (w1062:i32)
                  n551 = Increment(x=w1062) -> (x+1=w1059:i32)
                  n552 = Select(t=w1056, s=w1053, f=w1055) -> (s? t:f=w1054:dbl[])
                  n553 = Array Size(array=w1054) -> (size(s)=w1061:i32)
                  n554 = Less?(x=w1059, y=w1061) -> (x < y?=w1060:bool)
                  "Step Rate" <- w1060
                  n555 = case shown="False" w1060 {
                    tunnel: w1059 -> [_ w1092]
                    tunnel: w1052 -> [w1069 w1091]
                    tunnel: [w1068 w1091] -> w1058
                    tunnel: w1057 -> [w1067 _]
                    tunnel: w1053 -> [w1065 _]
                    frame False {
                      # "Step Temp?"
                      n556 = local read "Magnetic Field array (T)"() -> (w1064:dbl[])
                      n557 = local read "Temperature Array"() -> (w1066:dbl[])
                      n558 = local read "i"() -> (w1073:i32)
                      n559 = Select(t=w1064, s=w1065, f=w1066) -> (s? t:f=w1063:dbl[])
                      n560 = Increment(x=w1073) -> (x+1=w1071:i32)
                      n561 = local write "j"(0 ("f")) -> ()
                      n562 = Array Size(array=w1063) -> (size(s)=w1072:i32)
                      n563 = Less?(x=w1071, y=w1072) -> (x < y?=w1070:bool)
                      "Step Temp" <- w1070
                      n564 = case shown="True" w1070 {
                        tunnel: w1071 -> [_ w1090]
                        tunnel: w1069 -> [w1078 w1089]
                        tunnel: [w1077 w1089] -> w1068
                        tunnel: w1067 -> [w1076 _]
                        frame False {
                          # "Heater OFF"
                          # "Finished"
                          n565 = local write "i"(0 ("i")) -> ()
                          n566 = stacked-sequence {
                            tunnel: w1078 -> [w1082 _ _]
                            tunnel: [w1081 _ _] -> w1077
                            tunnel: w1076 -> [_ w1086 w1087]
                            frame #0 {
                              n567 = local read "Lake Shore"() -> (w1083:refnum<visa-resource-name>)
                              n568 = VISA Write(VISA resource name=w1083, write buffer="RANGE,1,0", error in (no error)=w1082) -> (error out=w1081:errorcluster)  [unwired: 2 out]
                            }
                            frame #1 {
                              n569 = call "ips_switchHeaterOff.vi"("Instrument address"=w1086, "Rate"=2.0) -> ()  [unwired: 1 out]
                            }
                            frame #2 {
                              n570 = call "GPIB - BusCommand.vi"("Command"="H0", "Address"=w1087) -> ()  [unwired: 2 out]
                            }
                          }
                          n571 = local write "Record ALL"(FALSE ("Record ALL")) -> ()
                          "Finished" <- TRUE
                        }
                        frame True {
                          n572 = local write "i"(w1090) -> ()
                        }
                      }
                    }
                    frame True {
                      n573 = local write "j"(w1092) -> ()
                    }
                  }
                }
                frame #3 {
                  # "Set rates"
                  n574 = local read "Temp/Magnetic Field"() -> (w1096:bool)
                  n575 = local read "Max count array"() -> (w1095:i32[])
                  n576 = local read "j"() -> (w1098:i32)
                  n577 = case shown="True" w1096 {
                    tunnel: w1099 -> [w1104 _]
                    tunnel: w1094 -> [w1100 w1111]
                    tunnel: [w1100 w1110] -> w1093
                    frame False {
                      n578 = local read "Sweep Rate Array"() -> (w1103:dbl[])
                      n579 = local read "j"() -> (w1102:i32)
                      n580 = Index Array(array=w1103, index=w1102) -> (element=w1101:dbl)
                      n581 = Number To Fractional String(number=w1101, precision (6)=i16 3) -> (F-format string=w1107:string)  [unwired: 2 in]
                      n582 = Concatenate Strings("T" ("format string"), w1107) -> (w1108:string)
                      n583 = call "GPIB - BusCommand.vi"("Command"=w1108, "Address"=w1104) -> ()  [unwired: 2 out]
                      n584 = local write "Sweep Rate (T/min)"(w1101) -> ()
                    }
                    frame True {
                      n585 = local read "T Sweep Rate Array"() -> (w1117:dbl[])
                      n586 = local read "j"() -> (w1118:i32)
                      n587 = Index Array(array=w1117, index=w1118) -> (element=w1113:dbl)
                      n588 = Number To Fractional String(number=w1113, precision (6)=i16 1) -> (F-format string=w1115:string)  [unwired: 2 in]
                      n589 = local read "Lake Shore"() -> (w1109:refnum<visa-resource-name>)
                      n590 = local write "Temp Ramping Rate (K/min)"(w1113) -> ()
                      n591 = Concatenate Strings("RAMP 1,1," ("string"), w1115) -> (w1116:string)
                      n592 = VISA Write(VISA resource name=w1109, write buffer=w1116, error in (no error)=w1111) -> (error out=w1110:errorcluster)  [unwired: 2 out]
                    }
                  }
                  n593 = Index Array(array=w1095, index=w1098) -> (element=w1097:i32)
                  n594 = local write "Max Countl"(w1097) -> ()
                }
                frame #4 {
                  # "Set temperature/Field"
                  n595 = local read "Temp/Magnetic Field"() -> (w1120:bool)
                  n596 = case shown="True" w1120 {
                    tunnel: [w1122 w1129] -> w1121
                    tunnel: w1119 -> [w1123 w1128]
                    frame True {
                      n597 = local read "Magnetic Field array (T)"() -> (w1126:dbl[])
                      n598 = local read "i"() -> (w1127:i32)
                      n599 = Index Array(array=w1126, index=w1127) -> (element=w1124:dbl)
                      n600 = call "Set_B.vi"("error in (no error)"=w1123, "address string"="25", "Set Field (T)"=w1124) -> ("error out"=w1122:errorcluster)  [unwired: 8 in]
                    }
                    frame False {
                      n601 = local read "Temperature Array"() -> (w1132:dbl[])
                      n602 = local read "i"() -> (w1131:i32)
                      n603 = Index Array(array=w1132, index=w1131) -> (element=w1130:dbl)
                      n604 = local read "Lake Shore"() -> (w1134:refnum<visa-resource-name>)
                      n605 = Number To Fractional String(number=w1130, precision (6)=i16 3) -> (F-format string=w1135:string)  [unwired: 2 in]
                      n606 = Concatenate Strings("SETP 1," ("write buffer"), w1135) -> (w1137:string)
                      n607 = VISA Write(VISA resource name=w1134, write buffer=w1137, error in (no error)=w1128) -> (error out=w1129:errorcluster)  [unwired: 2 out]
                    }
                  }
                }
                frame #5 {
                  n608 = local read "Finished"() -> (w1140:bool)
                  n609 = case shown="False" w1140 {
                    tunnel: [w1169 w1202] -> w1141
                    tunnel: w1139 -> [_ _]
                    tunnel: w1138 -> [w1166 w1202]
                    frame False {
                      w1164 = "_" ("string")
                      # "Wait, create Files"
                      n610 = local read "Magnetic Field array (T)"() -> (w1151:dbl[])
                      n611 = local read "Temp/Magnetic Field"() -> (w1143:bool)
                      n612 = local read "Temperature Array"() -> (w1156:dbl[])
                      n613 = local read "T Sweep Rate Array"() -> (w1153:dbl[])
                      n614 = local read "Sweep Rate Array"() -> (w1154:dbl[])
                      n615 = local read "i"() -> (w1192:i32)
                      n616 = local read "j"() -> (w1190:i32)
                      n617 = Select(t=w1153, s=w1143, f=w1154) -> (s? t:f=w1152:dbl[])
                      n618 = Index Array(array=w1152, index=w1190) -> (element=w1161:dbl)
                      n619 = Round Toward -Infinity(1:w1161) -> (0:w1162:dbl)
                      n620 = Multiply(x=w1151, y=i16 1000 ("precision (6)")) -> (x*y=w1149:dbl[])
                      n621 = Select(t=w1149, s=w1143, f=w1156) -> (s? t:f=w1155:dbl[])
                      n622 = Index Array(array=w1155, index=w1192) -> (element=w1191:dbl)
                      n623 = Number To Fractional String(use system decimal point (T)=TRUE, number=w1191, precision (6)=i16 1) -> (F-format string=w1193:string)  [unwired: 1 in]
                      n624 = Subtract(x=w1161, y=w1162) -> (x-y=w1163:dbl)
                      n625 = Equal To 0?(x=w1163) -> (x = 0?=w1160:bool)
                      n626 = Select(t="mT" ("string"), s=w1143, f="K" ("string")) -> (s? t:f=w1146:string)
                      n627 = Select(t=i16 0 ("precision (6)"), s=w1160, f=i16 2 ("precision (6)")) -> (s? t:f=w1157:i16)
                      n628 = Number To Fractional String(use system decimal point (T)=TRUE, number=w1161, precision (6)=w1157) -> (F-format string=w1165:string)  [unwired: 1 in]
                      n629 = Select(t="Kpm" ("string"), s=w1143, f="Tpm" ("string")) -> (s? t:f=w1142:string)
                      n630 = Concatenate Strings("Directory", "\\" ("string"), "FileName", w1164, w1193, w1146, w1164, w1165, w1142) -> (w1186:string)
                      n631 = Search and Replace String(replace all?=TRUE ("replace all? (F)"), input string=w1186, search string=".", replace string="p" ("substring (\"\")"), error in=w1166) -> (result string=w1181:string, error out=w1176:errorcluster)  [unwired: 3 in, 2 out]
                      n632 = local write "Step Rate"(FALSE ("Step Rate")) -> ()
                      n633 = Concatenate Strings(w1181, ".txt" ("string")) -> (w1180:string)
                      n634 = local read "Step Temp"() -> (w1170:bool)
                      n635 = String To Path(string=w1180) -> (path=w1179:path)
                      n636 = Open/Create/Replace File(file path (use dialog)=w1179, error in=w1176, operation (0:open)=T5."open or create") -> (refnum out=w1168:refnum<file>, error out=w1169:errorcluster)  [unwired: 3 in, 1 out]
                      n637 = local write "refnum out"(w1168) -> ()
                      n638 = Refnum to Path(1:w1168) -> (0:w1171:path)
                      n639 = call "Create_sweep_files.vi"("Measurement File"=w1171) -> ("Path 3"=w1174:path, "Path 2"=w1173:path, "Path"=w1172:path)  [unwired: 8 in]
                      n640 = local write "Measurement File"(w1171) -> ()
                      n641 = case shown="True" w1170 {
                        frame False {
                        }
                        frame True {
                          n642 = Get Date/Time In Seconds() -> (seconds since 1Jan1904=w1195:timestamp)
                          n643 = local write "Step Temp"(FALSE ("Step Temp")) -> ()
                          n644 = while {
                            tunnel: w1195 -> [w1200]
                            stop <- w1197 stop-if-true
                            n645 = Get Date/Time In Seconds() -> (seconds since 1Jan1904=w1201:timestamp)
                            n646 = Subtract(x=w1201, y=w1200) -> (x-y=w1199:dbl)
                            "Wait (s)" <- w1199
                            n647 = Greater Or Equal?(x=w1199, y="secs to wait") -> (x >= y?=w1197:bool)
                          }
                        }
                      }
                      n648 = local write "Measurement File_dn"(w1174) -> ()
                      n649 = local write "Measurement File_average"(w1172) -> ()
                      n650 = local write "Measurement File_up"(w1173) -> ()
                    }
                    frame True {
                    }
                  }
                }
                frame #6 {
                  n651 = local read "Finished"() -> (w1203:bool)
                  n652 = case shown="True" w1203 {
                    frame False {
                      n653 = local write "Measuring"(TRUE ("Measuring")) -> ()
                    }
                    frame True {
                      n654 = local write "Measure /Pause"(FALSE ("Measure /Pause")) -> ()
                    }
                  }
                }
              }
            }
            frame "Return" {
            }
          }
        }
      }
      frame Error {
        # "Return true for any case which should stop the loop."
      }
    }
  }
  n655 = VISA Read(VISA resource name=w31, byte count=u32 100, error in (no error)=w33) -> (VISA resource name out=w30:refnum<visa-resource-name>, read buffer=w29:string, error out=w32:errorcluster)  [unwired: 1 out]
  n656 = VISA Open(error in (no error)=w32, VISA resource name="Magnetic Field") -> (VISA resource name=w120:refnum<visa-resource-name>, error out=w102:errorcluster)  [unwired: 3 in]
  n657 = VISA Open(error in (no error)=w102, VISA resource name="Lake Shore") -> (VISA resource name=w97:refnum<visa-resource-name>, error out=w69:errorcluster)  [unwired: 3 in]
  n658 = VISA Write(VISA resource name="Lake Shore", write buffer="KRDG?a", error in (no error)=w69) -> (VISA resource name out=w66:refnum<visa-resource-name>, error out=w65:errorcluster)  [unwired: 1 out]
  n659 = VISA Read(VISA resource name=w66, byte count=w72, error in (no error)=w65) -> (VISA resource name out=w63:refnum<visa-resource-name>, read buffer=w77:string, error out=w64:errorcluster)  [unwired: 1 out]
  n660 = VISA Write(VISA resource name=w63, write buffer="SETP?a", error in (no error)=w64) -> (VISA resource name out=w62:refnum<visa-resource-name>, error out=w61:errorcluster)  [unwired: 1 out]
  n661 = VISA Read(VISA resource name=w62, byte count=w72, error in (no error)=w61) -> (VISA resource name out=w59:refnum<visa-resource-name>, read buffer=w76:string, error out=w60:errorcluster)  [unwired: 1 out]
  n662 = VISA Write(VISA resource name=w59, write buffer="RANGE?a", error in (no error)=w60) -> (VISA resource name out=w57:refnum<visa-resource-name>, error out=w58:errorcluster)  [unwired: 1 out]
  n663 = Fract/Exp String To Number(string=w77) -> (number=w75:dbl)  [unwired: 3 in, 1 out]
  n664 = VISA Read(VISA resource name=w57, byte count=w72, error in (no error)=w58) -> (read buffer=w71:string, error out=w68:errorcluster)  [unwired: 2 out]
  n665 = Fract/Exp String To Number(string=w76) -> (number=w74:dbl)  [unwired: 3 in, 1 out]
  n666 = Fract/Exp String To Number(string=w71) -> (number=w67:dbl)  [unwired: 3 in, 1 out]
  n667 = local write "Actual Temperature (K)"(w75) -> ()
  n668 = local write "Setpoint Temperature (K)"(w74) -> ()
  n669 = local write "Heater Range"(w67) -> ()
  n670 = case shown="True" w82 {
    frame False {
    }
    frame True {
      n671 = invoke on="I(B) 3" class="XYGraph (strict)" method="Reinit To Default"() -> ()  [unwired: 3 in, 3 out]
      n672 = invoke on="I(B) /Averaged/" class="XYGraph (strict)" method="Reinit To Default"() -> ()  [unwired: 3 in, 3 out]
      n673 = invoke on="P(T)" class="XYGraph (strict)" method="Reinit To Default"() -> ()  [unwired: 3 in, 3 out]
      n674 = invoke on="P(B)" class="XYGraph (strict)" method="Reinit To Default"() -> ()  [unwired: 3 in, 3 out]
      n675 = invoke on="I(T)" class="XYGraph (strict)" method="Reinit To Default"() -> ()  [unwired: 3 in, 3 out]
      n676 = invoke on="P(B) /Averaged/" class="XYGraph (strict)" method="Reinit To Default"() -> ()  [unwired: 3 in, 3 out]
    }
  }
  n677 = Decimal String To Number(string=w29) -> (number=w28:i32)  [unwired: 2 in, 1 out]
  n678 = local write "Keithley (IV conv) averaging"(w28) -> ()
  n679 = local read "Stepping Mode"() -> (w8:bool)
  n680 = while {
    shift-right: [w1234] -> w118
    shift-left: w99 -> [w1235]
    shift-right: [w1236] -> w123
    shift-left: w124 -> [w1237]
    tunnel: w30 -> [w1233]
    tunnel: w120 -> [w1232]
    tunnel: w68 -> [_]
    tunnel: [w1226] -> _
    tunnel: w107 -> [w1225]
    tunnel: w97 -> [w1224]
    tunnel: w38 -> [w1223]
    stop <- "stop" stop-if-true
    n681 = event shown="[10] \"Calibrate\": Value Change" {
      selector: _ -> [_ _ _ _ _ _ _ _ _ _ _ _ _ _ _ _]
      dyn-events: _ -> [_ _ _ _ _ _ _ _ _ _ _ _ _ _ _ _]
      timeout: 10 -> [_ _ _ _ _ _ _ _ _ _ _ _ _ _ _ _]
      tunnel: w1237 -> [w1247 w1293 w1311 w1321 w1335 w1406 w1410 w1414 w1470 w1486 w1503 w1546 w1563 w1587 w1589 w1600]
      tunnel: [w1246 w1293 w1311 w1321 w1335 w1406 w1410 w1414 w1470 w1486 w1503 w1546 w1563 w1587 w1589 w1600] -> w1236
      tunnel: w1235 -> [w1245 w1302 w1310 w1320 w1333 w1405 w1412 w1416 w1471 w1485 w1502 w1547 w1565 w1581 w1593 w1602]
      tunnel: [w1244 w1294 w1310 w1320 w1332 w1407 w1412 w1415 _ w1485 w1502 w1547 w1564 w1580 w1592 w1601] -> w1234
      tunnel: w1233 -> [w1243 w1303 _ _ _ _ _ _ _ _ _ _ _ _ _ _]
      tunnel: w1232 -> [w1242 _ _ _ _ _ _ _ _ _ _ _ _ _ _ _]
      tunnel: [w1240 w1292 w1309 w1319 w1334 w1408 w1411 w1413 w1469 w1484 w1501 w1545 w1562 w1588 w1590 _] -> w1226
      tunnel: w1225 -> [w1240 w1292 w1309 w1322 w1334 w1408 w1411 w1413 w1469 w1484 w1501 w1545 w1562 w1588 w1590 _]
      tunnel: w1224 -> [_ _ _ _ _ _ _ _ _ _ _ _ w1566 w1579 w1594 w1599]
      tunnel: [_ _ _ _ _ _ _ _ w1471 _ _ _ _ _ _ _] -> _
      tunnel: w1223 -> [w1239 _ _ _ _ _ _ _ _ _ _ _ _ _ _ _]
      event Timeout {
        n682 = event-data() -> ()  [unwired: 1 in, 3 out]
        n683 = case shown="True" "Measuring" {
          tunnel: w1247 -> [w1249 w1272]
          tunnel: [w1249 w1271] -> w1246
          tunnel: w1245 -> [w1248 w1250]
          tunnel: [w1248 w1270] -> w1244
          tunnel: w1243 -> [_ w1263]
          tunnel: w1242 -> [_ w1262]
          tunnel: w1239 -> [_ w1253]
          frame False {
          }
          frame True {
            w1261 = ":FETCh? " ("data")
            w1264 = u32 1000 ("byte count")
            # "Generate the data here."
            n684 = case shown="No Error" w1250 {
              selector: w1250 -> [w1284 w1285]
              tunnel: [w1284 w1285] -> w1258
              tunnel: [w1283 _] -> w1257
              frame No Error {
                n685 = Get Date/Time In Seconds() -> (seconds since 1Jan1904=w1283:timestamp)
              }
              frame Error {
              }
            }
            n686 = VISA Write(VISA resource name=w1263, write buffer=w1261, error in (no error)=w1258) -> (VISA resource name out=w1269:refnum<visa-resource-name>, error out=w1267:errorcluster)  [unwired: 1 out]
            n687 = VISA Write(VISA resource name=w1262, write buffer=w1261, error in (no error)=w1267) -> (VISA resource name out=w1268:refnum<visa-resource-name>, error out=w1266:errorcluster)  [unwired: 1 out]
            n688 = VISA Read(VISA resource name=w1269, byte count=w1264, error in (no error)=w1266) -> (read buffer=w1259:string, error out=w1265:errorcluster)  [unwired: 2 out]
            n689 = VISA Read(VISA resource name=w1268, byte count=w1264, error in (no error)=w1265) -> (read buffer=w1260:string, error out=w1255:errorcluster)  [unwired: 2 out]
            n690 = case shown="False" "DaQ" {
              tunnel: w1255 -> [w1274 w1280]
              tunnel: [w1274 w1279] -> w1254
              tunnel: w1253 -> [_ w1278]
              tunnel: [0.0 ("Output") w1276] -> w1251
              frame False {
              }
              frame True {
                n691 = local read "Number of Samples"() -> (w1282:i32)
                n692 = call-poly <vilib>:"DAQmx Read.vi"("task/channels in"=w1278, "number of samples per channel"=w1282, "error in"=w1280) -> ("data"=w1281:dbl[], "error out"=w1279:errorcluster)  [unwired: 10 in, 1 out]
                n693 = call-poly <vilib>:"Mean.vi"("X"=w1281) -> ("mean"=w1277:dbl)  [unwired: 1 out]
                "Actual mean" <- w1277
                n694 = call "N Point Running Average.vi"("n"="Moving average", "Input"=w1277) -> ("Output"=w1276:dbl)
              }
            }
            n695 = Bundle("seconds since 1Jan1904"=w1257, "read buffer"=w1259, "read buffer"=w1260, "Output"=w1251) -> (w1256:T4)  [unwired: 1 in]
            n696 = Enqueue Element(queue=w1272, element=w1256, error in (no error)=w1254) -> (queue out=w1271:refnum<queue>, error out=w1270:errorcluster)  [unwired: 1 in, 1 out]
          }
        }
      }
      event "Keithley (IV conv) averaging": Value Change {
        n697 = event-data() -> ()  [unwired: 1 in, 6 out]
        n698 = Number To Decimal String(number="Keithley (IV conv) averaging") -> (decimal integer string=w1300:string)  [unwired: 1 in]
        n699 = Concatenate Strings("VOLTage:DC:AVERage:COUNt " ("write buffer"), w1300) -> (w1299:string)
        n700 = VISA Write(VISA resource name=w1303, write buffer=w1299, error in (no error)=w1302) -> (VISA resource name out=w1298:refnum<visa-resource-name>, error out=w1296:errorcluster)  [unwired: 1 out]
        n701 = VISA Write(VISA resource name=w1298, write buffer="VOLTage:DC:AVERage:COUNt?", error in (no error)=w1296) -> (VISA resource name out=w1291:refnum<visa-resource-name>, error out=w1295:errorcluster)  [unwired: 1 out]
        n702 = VISA Read(VISA resource name=w1291, byte count=u32 100, error in (no error)=w1295) -> (read buffer=w1289:string, error out=w1294:errorcluster)  [unwired: 2 out]
        n703 = Decimal String To Number(string=w1289) -> (number=w1288:i32)  [unwired: 2 in, 1 out]
        n704 = Equal?(x="Keithley (IV conv) averaging", y=w1288) -> (x = y?=→"Confirm":bool)
      }
      event "Max Field (T)": Value Change {
        n705 = event-data() -> ()  [unwired: 1 in, 6 out]
        n706 = Divide(x="Max Field (T)", y="dB (T)") -> (x/y=w1306:dbl)
        n707 = for {
          N: w1306 -> [_]
          tunnel: "dB (T)" -> [w1316]
          tunnel: [w1313] -> w1305 mode=indexing
          tunnel: "Min Field (T)" -> [w1314]
          tunnel: [0.0] -> _ mode=indexing
          i -> [w1317]
          n708 = Multiply(x=w1317, y=w1316) -> (x*y=w1315:dbl)
          n709 = Add(x=w1315, y=w1314) -> (x+y=w1313:dbl)
        }
        "B array" <- w1305
      }
      event "Sweep Rate (T/min)": Value Change {
        n710 = event-data() -> ("NewVal"=w1323:dbl)  [unwired: 1 in, 5 out]
        n711 = local read "Magnet"() -> (w1318:bool)
        n712 = case shown="False" w1318 {
          tunnel: w1323 -> [_ w1330]
          tunnel: w1322 -> [w1324 w1326]
          tunnel: [w1324 w1325] -> w1319
          frame False {
          }
          frame True {
            n713 = Number To Fractional String(number=w1330, precision (6)=i16 3) -> (F-format string=w1328:string)  [unwired: 2 in]
            n714 = Concatenate Strings("T" ("format string"), w1328) -> (w1327:string)
            n715 = call "GPIB - BusCommand.vi"("Command"=w1327, "Address"=w1326) -> ("Address(thru)"=w1325:T6)  [unwired: 1 out]
          }
        }
      }
      event "Field To Zero": Value Change {
        n716 = event-data() -> ()  [unwired: 1 in, 6 out]
        n717 = Two Button Dialog(message="Do you want to switch off the field?", 1:"No" ("F button name (\"Cancel\")"), 2:"Yes" ("T button name (\"OK\")")) -> (T button?=w1339:bool)
        n718 = case shown="True" w1339 {
          tunnel: w1334 -> [_ w1344]
          tunnel: w1333 -> [w1340 w1342]
          tunnel: [w1340 w1341] -> w1332
          frame False {
          }
          frame True {
            n719 = local read "Magnet"() -> (w1343:bool)
            n720 = case shown="False" w1343 {
              tunnel: w1344 -> [_ w1396]
              tunnel: w1342 -> [w1347 w1393]
              tunnel: [w1346 w1393] -> w1341
              frame False {
                n721 = local read "Lock_in_Amplifier"() -> (w1345:refnum<visa-resource-name>)
                n722 = stacked-sequence {
                  seq-local: [w1350 _] -> [_ w1362]
                  seq-local: [w1348 _] -> [_ w1359]
                  tunnel: w1347 -> [w1352 _]
                  tunnel: [_ w1365] -> w1346
                  tunnel: w1345 -> [w1349 w1360]
                  frame #0 {
                    n723 = VISA Write(VISA resource name=w1349, write buffer="AUXV?1", error in (no error)=w1352) -> (VISA resource name out=w1356:refnum<visa-resource-name>, error out=w1351:errorcluster)  [unwired: 1 out]
                    n724 = VISA Read(VISA resource name=w1356, byte count=u32 1000, error in (no error)=w1351) -> (read buffer=w1353:string, error out=w1350:errorcluster)  [unwired: 2 out]
                    n725 = Fract/Exp String To Number(string=w1353) -> (number=w1348:dbl)  [unwired: 3 in, 1 out]
                  }
                  frame #1 {
                    w1368 = 0.001 ("Voltage Step (V)")
                    n726 = local read "Sweep Rate (T/min)"() -> (w1367:dbl)
                    n727 = local read "V/I (Ohm)"() -> (w1364:dbl)
                    n728 = local read "B/V (T/V)"() -> (w1358:dbl)
                    n729 = xnode "Sweep Delay"("SweepRate"=w1367, "Resolution"=w1368, "BpV"=w1358) -> ("Result"=w1366:dbl)  [unwired: 1 in, 1 out]
                    n730 = call "Universal_Ramping.vi"("milliseconds to wait"=w1366, "Initial Voltage (V)"=w1359, "error in (no error)"=w1362, "Voltage Step (V)"=w1368, "Final Voltage (V)"=0.0, "VISA resource name"=w1360) -> ("error out"=w1365:errorcluster, "Actual Voltage (V)"=w1357:dbl)  [unwired: 3 in, 1 out]
                    n731 = local write "Actual Voltage (V)"(w1357) -> ()
                    n732 = xnode "AUXtoB"("BpV"=w1358, "Rm"=w1364, "Aux"=w1357) -> ("Result"=w1363:dbl)  [unwired: 1 in, 1 out]
                    n733 = local write "Actual B Field (T)"(w1363) -> ()
                  }
                }
              }
              frame True {
                n734 = local read "Sweep Rate (T/min)"() -> (w1395:dbl)
                n735 = call "ips_switchHeaterOff.vi"("Instrument address"=w1396, "Rate"=w1395) -> ("B"=w1394:dbl)
                n736 = local write "Actual Field (T)"(w1394) -> ()
              }
            }
          }
        }
      }
      event "Go to Set": Value Change {
        n737 = event-data() -> ()  [unwired: 1 in, 6 out]
        n738 = local read "V/I (Ohm)"() -> (w1403:dbl)
        n739 = local read "B/V (T/V)"() -> (w1402:dbl)
        n740 = local read "Lock_in_Amplifier"() -> (w1399:refnum<visa-resource-name>)
        n741 = local read "Sweep Rate (T/min)"() -> (w1401:dbl)
        n742 = local read "Magnet"() -> (w1404:bool)
        n743 = call "Ramp_Field.vi"("Set Field (T) in"="Set Field (T)", "Sweep Rate (T/min)"=w1401, "V/I (Ohm)"=w1403, "error in (no error)"=w1405, "Magnet"=w1404, "B/V (T/V)"=w1402, "VISA Refnum in"=w1399) -> ("error out"=w1407:errorcluster, "Actual Voltage (V)"=w1397:dbl, "Set Field (T) out"=w1400:dbl)  [unwired: 2 in]
        n744 = local write "Actual B Field (T)"(w1400) -> ()
        n745 = local write "Actual Voltage (V)"(w1397) -> ()
      }
      event "Measure /Pause": Value Change {
        n746 = event-data() -> ("NewVal"=w1409:bool)  [unwired: 1 in, 5 out]
        n747 = local write "Measuring"(w1409) -> ()
      }
      event "Stop": Value Change {
        n748 = event-data() -> ()  [unwired: 1 in, 6 out]
        n749 = local read "Measuring"() -> (w1417:bool)
        n750 = case shown="True" w1417 {
          tunnel: w1416 -> [w1418 w1420]
          tunnel: [w1418 w1421] -> w1415
          frame False {
          }
          frame True {
            w1422 = FALSE ("Measuring")
            n751 = local read "Temp/Magnetic Field"() -> (w1419:bool)
            n752 = local read "SaveSweep"() -> (w1423:bool)
            n753 = local write "Measuring"(w1422) -> ()
            n754 = local write "Measure /Pause"(w1422) -> ()
            n755 = case shown="False" w1419 {
              tunnel: [w1427 w1436] -> w1421
              tunnel: w1420 -> [w1426 w1437]
              frame False {
                n756 = local read "Lock_in_Amplifier"() -> (w1428:refnum<visa-resource-name>)
                n757 = local read "V/I (Ohm)"() -> (w1432:dbl)
                n758 = local read "Sweep Rate (T/min)"() -> (w1431:dbl)
                n759 = local read "Set Field (T)"() -> (w1433:dbl)
                n760 = local read "B/V (T/V)"() -> (w1429:dbl)
                n761 = local read "Magnet"() -> (w1430:bool)
                n762 = call "Ramp_Field.vi"("Set Field (T) in"=w1433, "Sweep Rate (T/min)"=w1431, "V/I (Ohm)"=w1432, "error in (no error)"=w1426, "Magnet"=w1430, "B/V (T/V)"=w1429, "VISA Refnum in"=w1428) -> ("error out"=w1427:errorcluster, "Actual Voltage (V)"=w1424:dbl, "Set Field (T) out"=w1425:dbl)  [unwired: 2 in]
                n763 = local write "Actual B Field (T)"(w1425) -> ()
                n764 = local write "Actual Voltage (V)"(w1424) -> ()
              }
              frame True {
                n765 = local read "Set temperature (K)"() -> (w1434:dbl)
                n766 = Number To Fractional String(number=w1434, precision (6)=i16 3) -> (F-format string=w1440:string)  [unwired: 2 in]
                n767 = local read "Lake Shore"() -> (w1435:refnum<visa-resource-name>)
                n768 = Concatenate Strings("SETP 1," ("write buffer"), w1440) -> (w1438:string)
                n769 = VISA Write(VISA resource name=w1435, write buffer=w1438, error in (no error)=w1437) -> (error out=w1436:errorcluster)  [unwired: 2 out]
              }
            }
            n770 = case shown="True" w1423 {
              tunnel: w1419 -> [_ w1442]
              frame False {
              }
              frame True {
                w1449 = 1 ("index (row)")
                w1450 = 0 ("index (row)")
                n771 = case shown="True" w1442 {
                  tunnel: [w1466 w1468] -> w1460
                  tunnel: [w1465 w1467] -> w1443
                  frame True {
                    n772 = local read "Averaged P(T)"() -> (w1465:dbl[][])
                    n773 = local read "I(T) /Averaged/"() -> (w1466:cluster{"B array":dbl[], dbl[]}[])
                  }
                  frame False {
                    n774 = local read "Averaged P(B)"() -> (w1467:dbl[][])
                    n775 = local read "I(B) /Averaged/"() -> (w1468:cluster{"B array":dbl[], dbl[]}[])
                  }
                }
                n776 = local read "Measurement File_average"() -> (w1461:path)
                n777 = local read "Averaged dt"() -> (w1452:dbl[][])
                n778 = Index Array(array=w1452, index (row)=w1450) -> (element=w1451:dbl[])  [unwired: 1 in]
                n779 = Index Array(array=w1452, index (row)=w1449) -> (element=w1445:dbl[])  [unwired: 1 in]
                n780 = Index Array(array=w1460, index=1) -> (element=w1456:cluster{"B array":dbl[], dbl[]})
                n781 = Index Array(array=w1460, index=0) -> (element=w1457:cluster{"B array":dbl[], dbl[]})
                n782 = Unbundle(w1456) -> ("B array"=w1447:dbl[], w1446:dbl[])
                n783 = Unbundle(w1457) -> ("B array"=w1455:dbl[], w1454:dbl[])
                n784 = Index Array(array=w1443, index (row)=w1450) -> (element=w1448:dbl[])  [unwired: 1 in]
                n785 = Index Array(array=w1443, index (row)=w1449) -> (element=w1444:dbl[])  [unwired: 1 in]
                n786 = Build Array(w1455, w1454, w1451, w1448, w1447, w1446, w1445, w1444) -> (w1453:dbl[][])
                n787 = call-poly <vilib>:"Write Delimited Spreadsheet.vi"("file path (dialog if empty)"=w1461, "format (%.3f)"="%.5g", "2D data"=w1453, "append to file? (F)"=TRUE ("transpose? (F)"), "transpose? (F)"=TRUE ("append to file? (F)")) -> ()  [unwired: 9 in, 2 out]
              }
            }
          }
        }
      }
      event "Sweep": Value Change {
        n788 = event-data() -> ("NewVal"=w1472:bool)  [unwired: 1 in, 5 out]
        n789 = case shown="True" w1472 {
          frame False {
          }
          frame True {
            n790 = local read "Measurement File"() -> (w1473:path)
            n791 = Two Button Dialog(message="Do you want to create additional files for the sweeping measurements?" ("string"), 1:"No" ("F button name (\"Cancel\")"), 2:"Yes" ("T button name (\"OK\")")) -> (T button?=w1475:bool)
            n792 = case shown="True" w1475 {
              tunnel: w1473 -> [_ w1480]
              frame False {
                n793 = local write "SaveSweep"(FALSE ("SaveSweep")) -> ()
              }
              frame True {
                n794 = call "Create_sweep_files.vi"("Measurement File"=w1480) -> ("Path 3"=→"Measurement File_dn":path, "Path 2"=→"Measurement File_up":path, "Path"=→"Measurement File_average":path)  [unwired: 8 in]
                "SaveSweep" <- TRUE
              }
            }
          }
        }
      }
      event "Measure Noise": Value Change {
        n795 = event-data() -> ("NewVal"=w1487:bool)  [unwired: 1 in, 5 out]
        n796 = case shown="True" w1487 {
          frame False {
          }
          frame True {
            n797 = local read "Gain (V/A)"() -> (w1492:dbl)
            n798 = call "Noise_measurement.vi"("Gain (V/A)"=w1492, "Cycles"="Cycles", "Lower Cut-Off"="Cut-Off Frequency", "minimum value"="minimum value", "Filter On"="Filter On", "maximum value"="maximum value", "physical channels"="physical channels", "rate"="Rate", "samples per channel"="Samples per channel") -> ("Current (pA) Filtered"=→"Current (pA) Filtered":waveform(dbl), "PSD (pA/Hz^1/2) Peaks Removed"=→"PSD (pA/Hz^1/2) Peaks Removed":cluster{"f0":dbl, "df":dbl, "magnitude":dbl[]}, "Current (pA)"=→"Current (pA)":dbl[], "PSD (pA/Hz^1/2)"=→"PSD (pA/Hz^1/2)":cluster{"f0":dbl, "df":dbl, "magnitude":dbl[]})  [unwired: 3 in]
          }
        }
      }
      event "Calibrate": Value Change {
        n799 = event-data() -> ()  [unwired: 1 in, 6 out]
        n800 = case shown="True" "Calibrate" {
          frame False {
          }
          frame True {
            w1507 = dbl[] []
            n801 = while {
              shift-right: [w1540] -> w1505
              shift-left: dbl[][] [] -> [w1539]
              shift-right: [w1523] -> _
              shift-left: w1507 -> [w1535]
              shift-right: [w1532] -> _
              shift-left: w1507 -> [w1534]
              shift-right: [w1522] -> _
              shift-left: w1507 -> [w1533]
              shift-right: [w1514] -> _
              shift-left: 0.0 ("Set Field out") -> [w1513]
              stop <- w1536 stop-if-true
              n802 = call "Calibtarion.vi"("Dwell Time (ms)"="Dwell Time (ms)", "V array in (V)"=w1535, "I array in (A)"=w1533, "Collected array in"=w1539, "B array in (T)"=w1534, "Set Field (T)"=w1513, "dB"="dB") -> ("Best Linear Fit"=w1524:dbl[], "appended array"=→"appended array":dbl[][], "slope"=→"B/V (T/V)":dbl, "V array out (V)"=w1522:dbl[], "Boolean"=w1538:bool, "I array out (A)"=w1523:dbl[], "intercept 2"=→"I0 (A)":dbl, "Collected array out"=w1540:dbl[][], "intercept"=→"B0 (T)":dbl, "B array Out"=w1532:dbl[], "slope 2"=→"V/I (Ohm)":dbl, "Best Linear Fit 2"=w1529:dbl[], "Set Field out"=w1514:dbl)
              n803 = Bundle("V array out (V)"=w1522, "I array out (A)"=w1523) -> (w1531:T16)  [unwired: 1 in]
              n804 = Bundle("V array out (V)"=w1522, "Best Linear Fit"=w1524) -> (w1525:T17)  [unwired: 1 in]
              n805 = Bundle("I array out (A)"=w1523, "B array Out"=w1532) -> (w1527:T18)  [unwired: 1 in]
              n806 = Bundle("I array out (A)"=w1523, "Best Linear Fit 2"=w1529) -> (w1528:T19)  [unwired: 1 in]
              n807 = Or(x=w1538, y="stop 2") -> (x .or. y?=w1536:bool)
              n808 = Build Array(w1531, w1525) -> (→"V_I":T20)
              n809 = Build Array(w1527, w1528) -> (→"B_V":T21)
            }
            n810 = flat-sequence {
              tunnel: w1505 -> [w1511]
              frame #0 {
                n811 = Two Button Dialog(message="Do you want to save calibration file?") -> (T button?=w1510:bool)  [unwired: 2 in]
                n812 = case shown="True" w1510 {
                  tunnel: w1511 -> [_ w1512]
                  frame False {
                  }
                  frame True {
                    n813 = call-poly <vilib>:"Write Delimited Spreadsheet.vi"("2D data"=w1512) -> ()  [unwired: 13 in, 2 out]
                  }
                }
              }
            }
          }
        }
      }
      event "New Measurement File": Value Change {
        n814 = event-data() -> ()  [unwired: 1 in, 6 out]
        n815 = local read "Sweep"() -> (w1542:bool)
        n816 = Open/Create/Replace File(prompt="Please select measurement file\n", operation (0:open)=T5."replace or create with confirmation") -> (refnum out=w1548:refnum<file>)  [unwired: 4 in, 2 out]
        n817 = local write "refnum out"(w1548) -> ()
        n818 = Refnum to Path(1:w1548) -> (0:w1543:path)
        n819 = case shown="True" w1542 {
          tunnel: w1543 -> [_ w1551]
          frame False {
          }
          frame True {
            n820 = Two Button Dialog(message="Do you want to create additional files for the sweeping measurements?" ("string"), 1:"No" ("F button name (\"Cancel\")"), 2:"Yes" ("T button name (\"OK\")")) -> (T button?=w1553:bool)
            n821 = case shown="True" w1553 {
              tunnel: w1551 -> [_ w1561]
              frame False {
                n822 = local write "SaveSweep"(FALSE ("SaveSweep")) -> ()
              }
              frame True {
                n823 = call "Create_sweep_files.vi"("Measurement File"=w1561) -> ("Path 3"=w1558:path, "Path 2"=w1559:path, "Path"=w1560:path)  [unwired: 8 in]
                n824 = local write "Measurement File_dn"(w1558) -> ()
                n825 = local write "Measurement File_average"(w1560) -> ()
                n826 = local write "Measurement File_up"(w1559) -> ()
                n827 = local write "SaveSweep"(TRUE) -> ()
              }
            }
          }
        }
        n828 = local write "Measurement File"(w1543) -> ()
        n829 = local write "Offset?"(FALSE ("Offset?")) -> ()
        n830 = local write "First?"(TRUE ("First?")) -> ()
      }
      event "Heater On/Off": Value Change {
        n831 = event-data() -> ()  [unwired: 1 in, 6 out]
        n832 = case shown="False" "Heater On/Off" {
          tunnel: w1566 -> [w1571 w1577]
          tunnel: w1565 -> [w1569 w1578]
          tunnel: [w1568 w1576] -> w1564
          frame False {
            n833 = VISA Write(VISA resource name=w1571, write buffer="RANGE,1,0", error in (no error)=w1569) -> (error out=w1568:errorcluster)  [unwired: 2 out]
          }
          frame True {
            n834 = Number To Decimal String(number="Heater Range") -> (decimal integer string=w1574:string)  [unwired: 1 in]
            n835 = Concatenate Strings("RANGE,1," ("write buffer"), w1574) -> (w1572:string)
            n836 = VISA Write(VISA resource name=w1577, write buffer=w1572, error in (no error)=w1578) -> (error out=w1576:errorcluster)  [unwired: 2 out]
          }
        }
      }
      event "Set temperature (K)": Value Change {
        n837 = event-data() -> ()  [unwired: 1 in, 6 out]
        n838 = local read "Set temperature (K)"() -> (w1582:dbl)
        n839 = Number To Fractional String(number=w1582, precision (6)=i16 3) -> (F-format string=w1585:string)  [unwired: 2 in]
        n840 = Concatenate Strings("SETP 1," ("write buffer"), w1585) -> (w1583:string)
        n841 = VISA Write(VISA resource name=w1579, write buffer=w1583, error in (no error)=w1581) -> (error out=w1580:errorcluster)  [unwired: 2 out]
      }
      event "Temp Ramping Rate (K/min)": Value Change {
        n842 = event-data() -> ()  [unwired: 1 in, 6 out]
        n843 = local read "Temp Ramping Rate (K/min)"() -> (w1591:dbl)
        n844 = Number To Fractional String(number=w1591, precision (6)=i16 1) -> (F-format string=w1597:string)  [unwired: 2 in]
        n845 = Concatenate Strings("RAMP 1,1," ("string"), w1597) -> (w1596:string)
        n846 = VISA Write(VISA resource name=w1594, write buffer=w1596, error in (no error)=w1593) -> (error out=w1592:errorcluster)  [unwired: 2 out]
      }
      event "Heater Range": Value Change {
        n847 = event-data() -> ()  [unwired: 1 in, 6 out]
        n848 = local read "Heater On/Off"() -> (w1603:bool)
        n849 = case shown="True" w1603 {
          tunnel: w1602 -> [w1604 w1609]
          tunnel: [w1604 w1608] -> w1601
          tunnel: w1599 -> [_ w1607]
          frame False {
          }
          frame True {
            n850 = local read "Heater Range"() -> (w1605:enum16{"Off", "Low", "Medium", "High"})
            n851 = Number To Decimal String(number=w1605) -> (decimal integer string=w1611:string)  [unwired: 1 in]
            n852 = Concatenate Strings("RANGE,1," ("write buffer"), w1611) -> (w1610:string)
            n853 = VISA Write(VISA resource name=w1607, write buffer=w1610, error in (no error)=w1609) -> (error out=w1608:errorcluster)  [unwired: 2 out]
          }
        }
      }
    }
    n854 = Reciprocal(x="Sampling rate (Hz)") -> (1/x=w1230:dbl)
    n855 = Multiply(x=w1230, y=1000.0) -> (x*y=w1228:dbl)
    n856 = Wait Until Next ms Multiple(millisecond multiple=w1228) -> ()  [unwired: 1 out]
  }
  n857 = local read "Field Step (T)"() -> (w10:dbl)
  n858 = local read "Max Field (T)"() -> (w90:dbl)
  n859 = local read "dB (T)"() -> (w11:dbl)
  n860 = local read "Min Field (T)"() -> (w91:dbl)
  n861 = Select(t=w10, s=w8, f=w11) -> (s? t:f=w9:dbl)
  n862 = Divide(x=w90, y=w9) -> (x/y=w3:dbl)
  n863 = Increment(x=w3) -> (x+1=w2:dbl)
  n864 = for {
    N: w2 -> [_]
    tunnel: w9 -> [w1616]
    tunnel: [w1613] -> w53 mode=indexing
    tunnel: w91 -> [w1614]
    tunnel: [0.0] -> _ mode=indexing
    i -> [w1617]
    n865 = Multiply(x=w1617, y=w1616) -> (x*y=w1615:dbl)
    n866 = Add(x=w1615, y=w1614) -> (x+y=w1613:dbl)
  }
  n867 = Multiply(x=w53, y=0.0) -> (x*y=w50:dbl[])
  n868 = Array Size(array=w50) -> (size(s)=w1:i32)
  n869 = local write "B array"(w53) -> ()
  n870 = Array Subset(array=w50, length=w1) -> (w49:dbl[])  [unwired: 1 in]
  n871 = Build Array(w50, w50) -> (w51:dbl[][])
  n872 = local read "Max temperature (K)"() -> (w23:dbl)
  n873 = local read "Min Temperature (K)"() -> (w25:dbl)
  n874 = local write "Averaged I(B)"(w51) -> ()
  n875 = Build Array(w49, w49) -> (w4:dbl[][])
  "Stepped P(B)" <- w4
  n876 = Divide(x=w23, y="dt (K)") -> (x/y=w26:dbl)
  n877 = local write "Averaged P(B)"(w4) -> ()
  n878 = local write "Averaged dt"(w4) -> ()
  n879 = for {
    N: w26 -> [_]
    tunnel: "dt (K)" -> [w1622]
    tunnel: [w1619] -> w15 mode=indexing
    tunnel: w25 -> [w1620]
    tunnel: [0.0] -> _ mode=indexing
    i -> [w1623]
    n880 = Multiply(x=w1623, y=w1622) -> (x*y=w1621:dbl)
    n881 = Add(x=w1621, y=w1620) -> (x+y=w1619:dbl)
  }
  "T array" <- w15
  n882 = Multiply(x=w15, y=0.0) -> (x*y=w14:dbl[])
  n883 = Array Size(array=w14) -> (size(s)=w18:i32)
  n884 = Decrement(x=w18) -> (x-1=w19:i32)
  n885 = Array Subset(array=w14, length=w19) -> (w20:dbl[])  [unwired: 1 in]
  n886 = Build Array(w14, w14) -> (w17:dbl[][])
  n887 = local write "Averaged I(T)"(w17) -> ()
  n888 = Build Array(w20, w20) -> (w21:dbl[][])
  n889 = local write "Averaged P(T)"(w21) -> ()
  n890 = local write "Averaged dt"(w21) -> ()
  n891 = local read "Lake Shore"() -> (w100:refnum<visa-resource-name>)
  n892 = local read "IV converter"() -> (w116:refnum<visa-resource-name>)
  n893 = local read "Magnetic Field"() -> (w115:refnum<visa-resource-name>)
  n894 = VISA Close(VISA resource name=w116, error in (no error)=w118) -> (error out=w119:errorcluster)
  n895 = VISA Close(VISA resource name=w115, error in (no error)=w119) -> (error out=w117:errorcluster)
  n896 = Release Queue(queue=w123, error in (no error)=w117) -> (error out=w113:errorcluster)  [unwired: 1 in, 2 out]
  n897 = Merge Errors(w113, w112) -> (w114:errorcluster)
  n898 = VISA Close(VISA resource name=w100, error in (no error)=w114) -> (error out=w111:errorcluster)
  n899 = local read "refnum out"() -> (w109:refnum<file>)
  n900 = Close File(refnum=w109, error in=w111) -> (error out=w110:errorcluster)  [unwired: 1 out]
  n901 = call <vilib>:"Simple Error Handler.vi"("error in (no error)"=w110) -> ()  [unwired: 4 in, 5 out]
  "i" <- w83
  "j" <- w83
